vi "Main.vi"() -> ()   [LabVIEW 2013]
uses:
  <vilib>/Utility/miscctls.llb/LVFontTypeDef.ctl
  <vilib>/Utility/error.llb/DialogType.ctl
panel:
  out "Error BuvVIctrl":string[](array[string])
  in  "Num of Buvs":u8
  out "BuvCtrlVI_VIRef":refnum<vi>[](array[refnum])
  out "BuvNameArr":string[](array[string])
  out "Buv IP":string[](array[string])
  out "Buv con ID":refnum<k5>
  out "LoadPhase":bool
  in  "Tab Control":enum32{"ПОСТОЯННОГО ТОКА", "ИМПУЛЬСНЫЕ"}(tab)
  in  "List of channels":i32(listbox)
  in  "ReadFromFile":bool
  in  "WriteToFile":bool
  out "Дата":string
  out "Время":string
  in  "Comm. current inc":dbl=0.5 caption="А" min=0.0 max=72.0 step=0.25
  in  "Common curr. dec":bool
  in  "Common curr. inc":bool
  in  "ConnectAll":bool
  in  "DisconnectAll":bool
  in  "Set Output ON All":bool caption="ВЫХОДЫ ИСТОЧНИКОВ"
  out "текущий ист.":u8
  in  "SetCurrent":dbl min=0.0 max=72.0 step=0.1 format="%#.1g"
  in  "SetVoltage":dbl min=0.0 max=30.0 step=0.1 format="%#.1g"
  in  "SetCurrentB":bool
  in  "SetVoltageB":bool
  in  "SetOutputOffB":bool
  in  "SetOutputOnB":bool
  in  "ConnectChannel":bool
  in  "DisconnectChannel":bool
  in  "WriteToFile Buv":bool
  in  "ReadFromFile Buv":bool
  in  "NewBuvName":string caption="Имя"
  in  "NewBuvIP":string="172.16.21.xx" caption="IP"
  in  "DeleteBuv":bool caption="Удалить БУВ"
  in  "Quit":bool=TRUE
  in  "AddNewBuv":bool caption="Добавить БУВ"
  out "message event":string=" INSTRUCTIONS:\r\rNormal Use:  When using subVIs that incorporate the error in/error out (or error I/O) structure, place this handler where you want to inform the user of an error, typically at the end of the I/O data path, as the last action of the program.  If the error in error? is ERROR, the handler creates a message describing the error and its source.  If the type of dialog = 1 (default), the message is displayed to the user, who can only acknowedge it.  If the type = 2, the user can acknowledge the message or abort execution; aborting a program with active I/O is not recommended.  If the type = 0, no message is displayed; this is used to process the error programmatically, and the error out cluster elements are wired to individual terminals for that reason.  \r\rOther Use:\n\r\nlocal testing.  To test the error code of a subVI or function that does not have the error I/O structure, you can wire its error code and a source string to the local error code and error source inputs.  If error in error? indicates no error and error code is not equal to 0, the local code and source are substituted for the error in values, and error? is set TRUE (ERROR)."
  out "message upd":string=" INSTRUCTIONS:\r\rNormal Use:  When using subVIs that incorporate the error in/error out (or error I/O) structure, place this handler where you want to inform the user of an error, typically at the end of the I/O data path, as the last action of the program.  If the error in error? is ERROR, the handler creates a message describing the error and its source.  If the type of dialog = 1 (default), the message is displayed to the user, who can only acknowedge it.  If the type = 2, the user can acknowledge the message or abort execution; aborting a program with active I/O is not recommended.  If the type = 0, no message is displayed; this is used to process the error programmatically, and the error out cluster elements are wired to individual terminals for that reason.  \r\rOther Use:\n\r\nlocal testing.  To test the error code of a subVI or function that does not have the error I/O structure, you can wire its error code and a source string to the local error code and error source inputs.  If error in error? indicates no error and error code is not equal to 0, the local code and source are substituted for the error in values, and error? is set TRUE (ERROR)."
  in  "List of LU buw":i32(listbox)
  in  "SetCurrentAll":bool
  in  "SetVoltageAll":bool
  in  "Comm. voltage %":dbl caption="%" min=0.0 max=100.0 step=0.5
  in  "Common volt. dec":bool
  in  "Common volt. inc":bool
  in  "DeleteChannel":bool
  in  "AddChannel":bool
  out "CURRENTSET":dbl[](array[numeric])
  out "NAME":string[](array[string])
  out "ADRESS":string[](array[string])
  out "Measure_VI":refnum<vi>[](array[refnum])
  # "ЛИНЗЫ ЖЕСТКОЙ ФОКУСИРОВКИ"
  # "ВСЕ ИСТОЧНИКИ"
  # "ИСТОЧНИК №_"
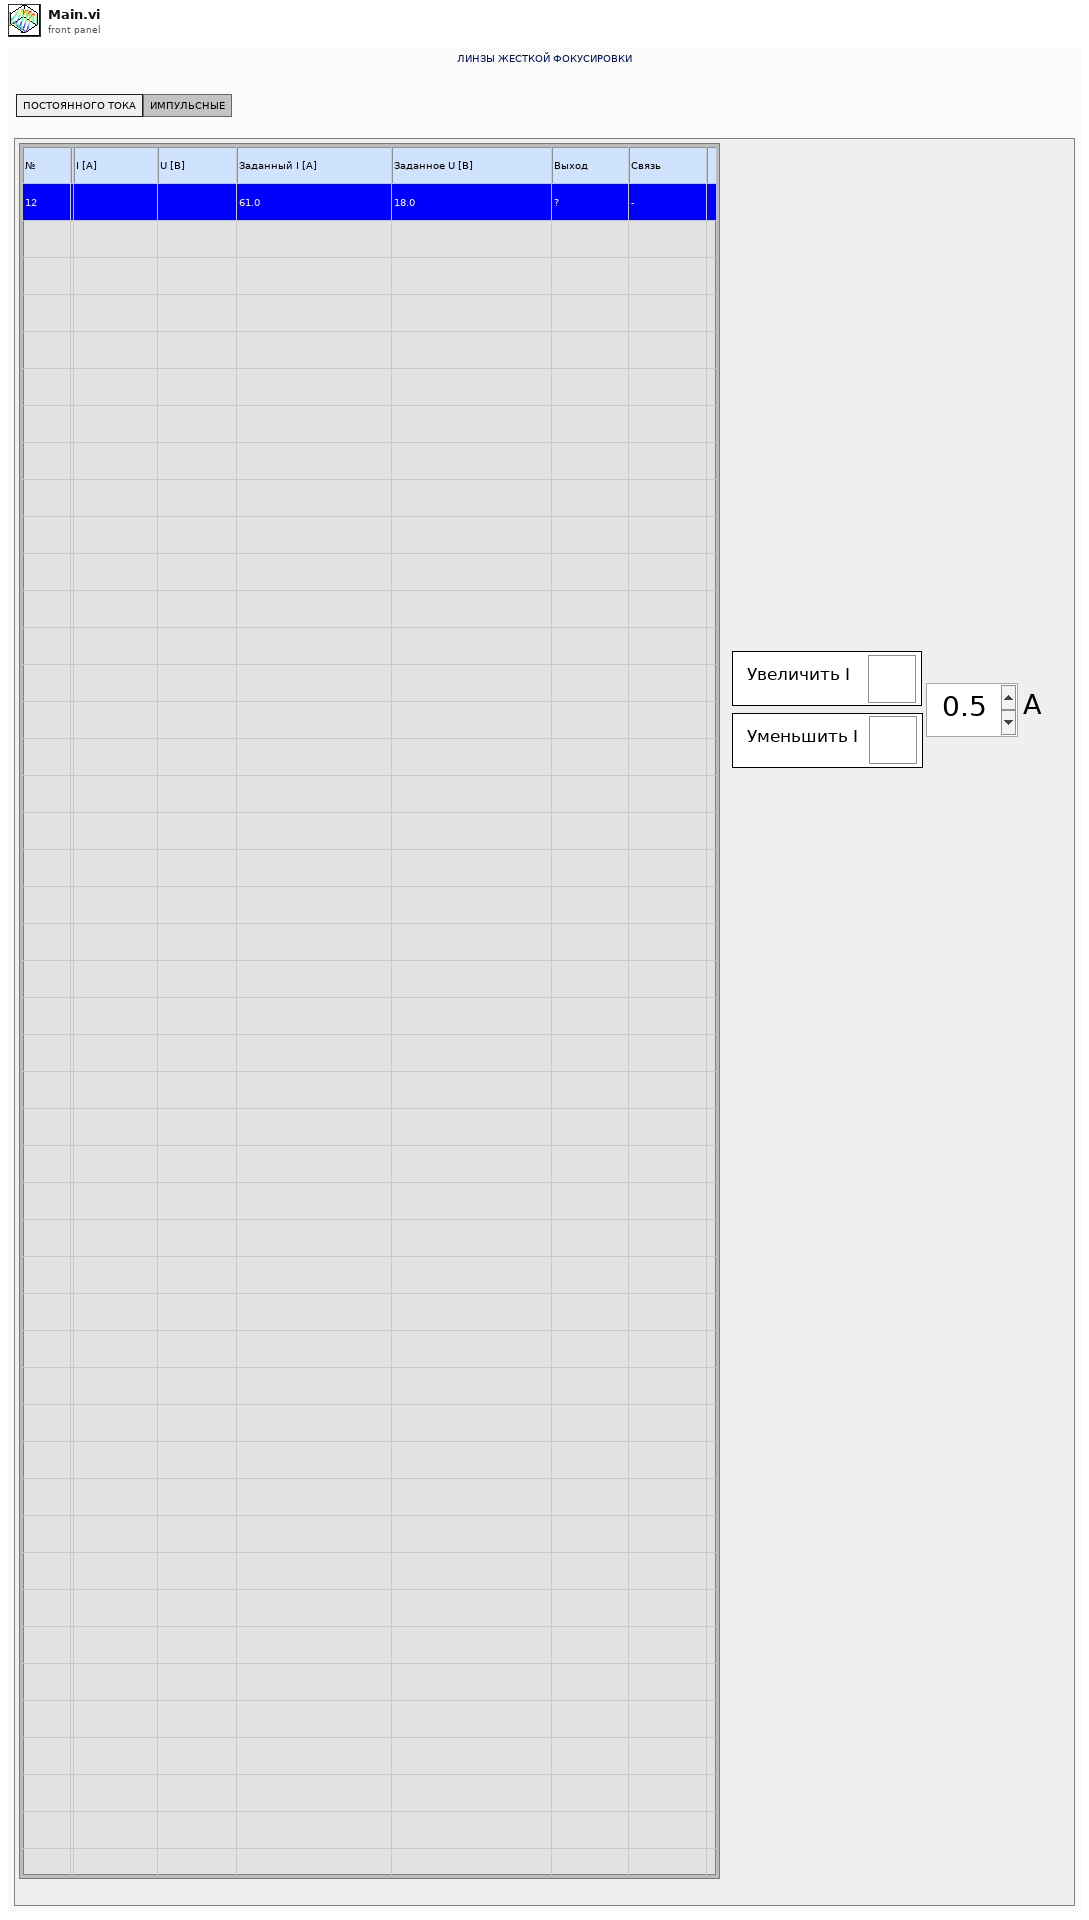
[diagram p1: front panel]
types:
  T1 = enum8{"Enabled", "Disabled", "Disabled and Grayed Out"}
  T2 = enum16{"open", "replace", "create", "open or create", "replace or create", "replace or create with confirmation"}
  T3 = typedef "DialogType.ctl" = u16
  T4 = typedef "LVFontTypeDef.ctl" = cluster{"Font Name":string, "Size":u16, "Bold":bool, "Italic":bool, "Underline":bool, "Strikeout":bool, "Color":u32}
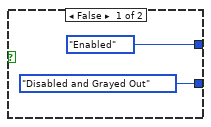
[diagram p3: hidden frame]
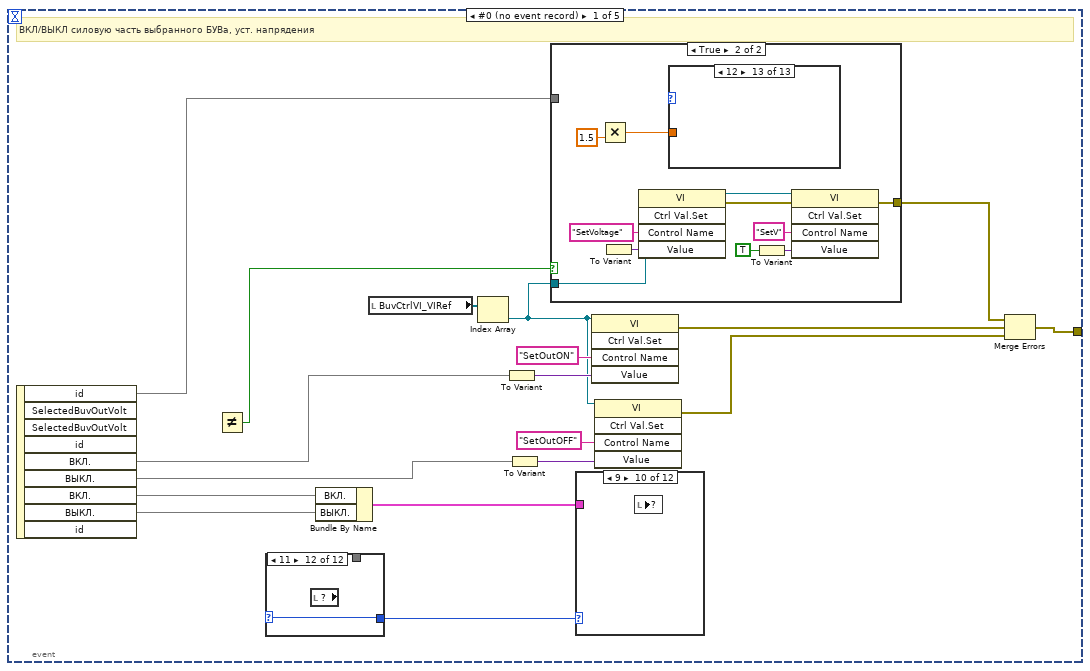
[diagram p4: hidden frame]
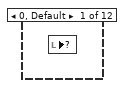
[diagram p5: hidden frame]
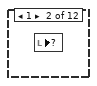
[diagram p6: hidden frame]
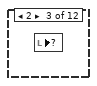
[diagram p7: hidden frame]
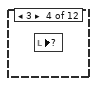
[diagram p8: hidden frame]
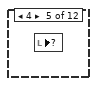
[diagram p9: hidden frame]
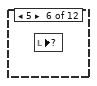
[diagram p10: hidden frame]
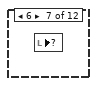
[diagram p11: hidden frame]
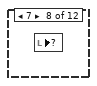
[diagram p12: hidden frame]
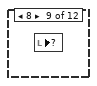
[diagram p13: hidden frame]
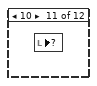
[diagram p14: hidden frame]
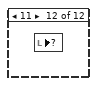
[diagram p15: hidden frame]
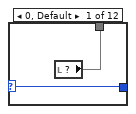
[diagram p16: hidden frame]
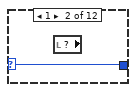
[diagram p17: hidden frame]
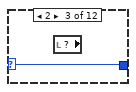
[diagram p18: hidden frame]
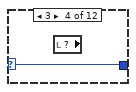
[diagram p19: hidden frame]
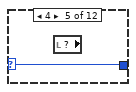
[diagram p20: hidden frame]
diagram:
  w2 = string[] [] ("GlobalInAdress")
  w5 = string[] [] ("GlobalInAdress")
  (unwired) T1."Enabled" ("Disabled")
  w21 = u8 0 ("Disabled")
  w6 = FALSE ("SetOutputOnB")
  w23 = FALSE ("OK Button")
  n1 = while {
    stop <- FALSE stop-if-true
    n2 = property on="List of channels" class="MCListbox (strict)"() -> ("ItemNames"=w34:string[][])  [unwired: 2 in, 2 out]
    n3 = Get Date/Time String(want seconds? (F)=TRUE) -> (date string=→"Дата":string, time string=→"Время":string)  [unwired: 2 in]
    n4 = Wait Until Next ms Multiple(millisecond multiple=u16 1000) -> ()  [unwired: 1 out]
    n5 = Empty Array?(array=w34) -> (empty?=w33:bool)
    n6 = case shown="True" w33 {
      tunnel: [T1."Enabled" ("Disabled") T1."Disabled and Grayed Out" ("Disabled")] -> w28
      frame False {
      }
      frame True {
      }
    }
    n7 = property on="Common curr. inc" class="Bool (strict)"("DisabledEnum"=w28) -> ()  [unwired: 2 in, 2 out]
    n8 = property on="Common curr. dec" class="Bool (strict)"("DisabledEnum"=w28) -> ()  [unwired: 2 in, 2 out]
    n9 = property on="Set Output ON All" class="Bool (strict)"("DisabledEnum"=w28) -> ()  [unwired: 2 in, 2 out]
    n10 = property on="Common volt. inc" class="Bool (strict)"("DisabledEnum"=w28) -> ()  [unwired: 2 in, 2 out]
    n11 = property on="DisconnectAll" class="Bool (strict)"("DisabledEnum"=w28) -> ()  [unwired: 2 in, 2 out]
    n12 = property on="SetVoltageB" class="Bool (strict)"("DisabledEnum"=w28) -> ()  [unwired: 2 in, 2 out]
    n13 = property on="ConnectChannel" class="Bool (strict)"("DisabledEnum"=w28) -> ()  [unwired: 2 in, 2 out]
    n14 = property on="SetOutputOnB" class="Bool (strict)"("DisabledEnum"=w28) -> ()  [unwired: 2 in, 2 out]
    n15 = property on="DisconnectChannel" class="Bool (strict)"("DisabledEnum"=w28) -> ()  [unwired: 2 in, 2 out]
    n16 = property on="SetOutputOffB" class="Bool (strict)"("DisabledEnum"=w28) -> ()  [unwired: 2 in, 2 out]
    n17 = property on="ConnectAll" class="Bool (strict)"("DisabledEnum"=w28) -> ()  [unwired: 2 in, 2 out]
    n18 = property on="SetCurrentB" class="Bool (strict)"("DisabledEnum"=w28) -> ()  [unwired: 2 in, 2 out]
  }
  n19 = while {
    stop <- FALSE stop-if-true
    n20 = property on="AddChannel" class="Bool (strict)"() -> ("Disabled"=w45:u8)  [unwired: 2 in, 2 out]
    n21 = Wait Until Next ms Multiple(millisecond multiple=u32 50) -> ()  [unwired: 1 out]
    n22 = local read "Quit"() -> (w43:bool)
    n23 = Not(x=w43) -> (.not. x?=w42:bool)
    n24 = Equal?(x=w45, y=u8 0) -> (x = y?=w41:bool)
    n25 = And(x=w42, y=w41) -> (x .and. y?=w40:bool)
    n26 = case shown="True" w40 {
      frame False {
      }
      frame True {
        w51 = string[] [] ("GlobalInAdress")
        n27 = local read "Measure_VI"() -> (w58:refnum<vi>[])
        n28 = Array Size(array=w58) -> (size(s)=w50:i32)
        n29 = for {
          N: w50 -> [_]
          tunnel: w58 -> [w121]
          shift-right: [w63] -> w49
          shift-left: w51 -> [w60]
          shift-right: [w62] -> w48
          shift-left: w51 -> [w61]
          shift-right: [w112] -> w46
          shift-left: w51 -> [w113]
          shift-right: [w103] -> w47
          shift-left: w51 -> [w108]
          shift-right: [w106] -> w54
          shift-left: w51 -> [w88]
          shift-right: [w101] -> w53
          shift-left: w51 -> [w102]
          i -> [w84]
          w100 = "" ("Control Name")
          n30 = Index Array(array=w121, index=w84) -> (element=w87:refnum<vi>)
          n31 = invoke on="Invoke Node" class="VI" method="Ctrl Val.Get"(reference=w87, "Control Name"="SetVoltageStr") -> (error out=w95:errorcluster, "Get Control Value Variant"=w111:variant)  [unwired: 2 in, 2 out]
          n32 = invoke class="VI" method="Ctrl Val.Get"(reference=w87, "Control Name"="SetCurrentStr") -> (error out=w94:errorcluster, "Get Control Value Variant"=w110:variant)  [unwired: 2 in, 2 out]
          n33 = invoke class="VI" method="Ctrl Val.Get"(reference=w87, "Control Name"="Error") -> (error out=w83:errorcluster, "Get Control Value Variant"=w89:variant)  [unwired: 2 in, 2 out]
          n34 = invoke class="VI" method="Ctrl Val.Get"(reference=w87, "Control Name"="GetCurrent") -> (error out=w97:errorcluster, "Get Control Value Variant"=w118:variant)  [unwired: 2 in, 2 out]
          n35 = invoke class="VI" method="Ctrl Val.Get"(reference=w87, "Control Name"="GetVoltage") -> (error out=w96:errorcluster, "Get Control Value Variant"=w119:variant)  [unwired: 2 in, 2 out]
          n36 = invoke class="VI" method="Ctrl Val.Get"(reference=w87, "Control Name"="Output") -> (error out=w93:errorcluster, "Get Control Value Variant"=w104:variant)  [unwired: 2 in, 2 out]
          n37 = Variant To Data(type=w100, Variant=w111) -> (data=w65:string)  [unwired: 1 in, 1 out]
          n38 = Variant To Data(type=w100, Variant=w110) -> (data=w70:string)  [unwired: 1 in, 1 out]
          n39 = Merge Errors(w83, w97, w96, w95) -> (w92:errorcluster)
          n40 = Variant To Data(type=w100, Variant=w118) -> (data=w115:string)  [unwired: 1 in, 1 out]
          n41 = Variant To Data(type=w100, Variant=w119) -> (data=w116:string)  [unwired: 1 in, 1 out]
          n42 = Variant To Data "Out"(type=w100, Variant=w104) -> (data=w90:string)  [unwired: 1 in, 1 out]
          n43 = Merge Errors(w94, w93) -> (w91:errorcluster)
          n44 = String Length(string=w65) -> (length=w66:i32)
          n45 = String Length(string=w70) -> (length=w73:i32)
          n46 = Variant To Data(type=FALSE, Variant=w89) -> (data=w59:bool)  [unwired: 1 in, 1 out]
          n47 = case shown="False" w59 {
            tunnel: w87 -> [_ w175]
            tunnel: w84 -> [w162 w168]
            tunnel: [w161 w166] -> w80
            frame False {
              n48 = Bundle(w162, "milliseconds to wait"=8) -> (w163:cluster{i32, "milliseconds to wait":i32})  [unwired: 1 in]
              n49 = property on="error" class="MCListbox (strict)"("ActiveCell"=w163, "CellBG"=u32 16777225) -> (error out=w161:errorcluster)  [unwired: 2 in, 1 out]
            }
            frame True {
              n50 = disable-structure shown="Enabled" {
                disable-tunnel: w175 -> [w191 w197]
                disable-tunnel: [w188 _] -> w171
                disable-tunnel: [w186 w197] -> w170
                disable-tunnel: [w184 _] -> w169
                disable-tunnel: w168 -> [w183 w198]
                disable-tunnel: [w182 w198] -> w167
                frame Disabled {
                  w185 = "Connect" ("Control Name")
                  n51 = invoke class="VI" method="Ctrl Val.Set"(reference=w191, "Control Name"=w185, "Value"=FALSE ("OK Button")) -> (reference out=w187:refnum<vi>, error out=w189:errorcluster)  [unwired: 2 in, 3 out]
                  n52 = flat-sequence {
                    tunnel: w189 -> [w196]
                    tunnel: [w196] -> w188
                    tunnel: w187 -> [w194]
                    tunnel: [w194] -> w186
                    tunnel: w185 -> [w193]
                    tunnel: [w193] -> w184
                    tunnel: w183 -> [w192]
                    tunnel: [w192] -> w182
                    frame #0 {
                      n53 = Wait (ms)(milliseconds to wait=u32 2000) -> ()  [unwired: 1 out]
                    }
                  }
                }
                frame Enabled {
                }
              }
              n54 = disable-structure shown="Enabled" {
                disable-tunnel: w171 -> [w179 w181]
                disable-tunnel: w170 -> [w178 _]
                disable-tunnel: w169 -> [w177 _]
                disable-tunnel: [w176 w181] -> w166
                frame Disabled {
                  n55 = invoke class="VI" method="Ctrl Val.Set"(reference=w178, error in=w179, "Control Name"=w177, "Value"=TRUE ("OK Button")) -> (error out=w176:errorcluster)  [unwired: 1 in, 4 out]
                }
                frame Enabled {
                }
              }
              n56 = Bundle(w167, "milliseconds to wait"=8) -> (w172:cluster{i32, "milliseconds to wait":i32})  [unwired: 1 in]
              n57 = property on="error" class="MCListbox (strict)"("ActiveCell"=w172, "CellBG"=u32 16711680) -> ()  [unwired: 2 in, 2 out]
            }
          }
          n58 = case shown="6, Default" w66 {
            tunnel: [4 ("milliseconds to wait") 5 ("milliseconds to wait")] -> w67
            tunnel: [0 ("milliseconds to wait") 0 ("milliseconds to wait")] -> w68
            frame 6, Default {
            }
            frame 7 {
            }
          }
          n59 = case shown="7" w73 {
            tunnel: [4 ("milliseconds to wait") 5 ("milliseconds to wait")] -> w72
            tunnel: [0 ("milliseconds to wait") 0 ("milliseconds to wait")] -> w71
            frame 6, Default {
            }
            frame 7 {
            }
          }
          n60 = Build Array (concatenate)(w60, w115) -> (w63:string[])
          n61 = Build Array (concatenate)(w61, w116) -> (w62:string[])
          n62 = Merge Errors(w92, w91, w80) -> (w86:errorcluster)
          n63 = call <vilib>:"General Error Handler.vi"("type of dialog (OK msg:1)"=u32 0 ("milliseconds to wait"), "error in (no error)"=w86) -> ()  [unwired: 9 in, 5 out]
          n64 = case shown="\"0\"" w90 {
            tunnel: ["+" ("Control Name") "" ("Control Name") "-" ("Control Name")] -> w82
            tunnel: w84 -> [w130 w135 w140]
            frame "1" {
              n65 = Bundle(w130, "milliseconds to wait"=6) -> (w132:cluster{i32, "milliseconds to wait":i32})  [unwired: 1 in]
              n66 = property on="out" class="MCListbox (strict)"("ActiveCell"=w132, "CellBG"=u32 5895331) -> ()  [unwired: 2 in, 2 out]
            }
            frame Default {
              n67 = Bundle(w135, "milliseconds to wait"=6) -> (w137:cluster{i32, "milliseconds to wait":i32})  [unwired: 1 in]
              n68 = property on="out" class="MCListbox (strict)"("ActiveCell"=w137, "CellBG"=u32 16777225) -> ()  [unwired: 2 in, 2 out]
            }
            frame "0" {
              n69 = Bundle(w140, "milliseconds to wait"=6) -> (w142:cluster{i32, "milliseconds to wait":i32})  [unwired: 1 in]
              n70 = property on="out" class="MCListbox (strict)"("ActiveCell"=w142, "CellBG"=u32 13816530) -> ()  [unwired: 2 in, 2 out]
            }
          }
          n71 = String Subset(string=w65, offset (0)=w68, length (rest)=w67) -> (substring=w64:string)
          n72 = String Subset(string=w70, offset (0)=w71, length (rest)=w72) -> (substring=w69:string)
          n73 = case shown="False" w59 {
            tunnel: ["+" ("Control Name") "-" ("Control Name")] -> w107
            tunnel: w84 -> [w146 w153]
            tunnel: w82 -> [w145 _]
            tunnel: [w145 "?" ("Control Name")] -> w81
            frame False {
              n74 = Bundle(w146, "milliseconds to wait"=7) -> (w148:cluster{i32, "milliseconds to wait":i32})  [unwired: 1 in]
              n75 = property on="active" class="MCListbox (strict)"("ActiveCell"=w148, "CellBG"=u32 5895331) -> ()  [unwired: 2 in, 2 out]
            }
            frame True {
              n76 = Bundle(w153, "milliseconds to wait"=7) -> (w159:cluster{i32, "milliseconds to wait":i32})  [unwired: 1 in]
              n77 = property on="active" class="MCListbox (strict)"("ActiveCell"=w159, "CellBG"=u32 14869218) -> (error out=w154:errorcluster)  [unwired: 2 in, 1 out]
              n78 = Bundle(w153, "milliseconds to wait"=6) -> (w152:cluster{i32, "milliseconds to wait":i32})  [unwired: 1 in]
              n79 = property on="out" class="MCListbox (strict)"(error in=w154, "ActiveCell"=w152, "CellBG"=u32 14869218) -> ()  [unwired: 1 in, 2 out]
            }
          }
          n80 = Search and Replace String(input string=w64, search string=",", replace string="." ("replace string (\"\")")) -> (result string=w77:string)  [unwired: 5 in, 3 out]
          n81 = Search and Replace String(input string=w69, search string=",", replace string="." ("replace string (\"\")")) -> (result string=w75:string)  [unwired: 5 in, 3 out]
          n82 = Build Array (concatenate)(w108, w75) -> (w103:string[])
          n83 = Build Array (concatenate)(w113, w77) -> (w112:string[])
          n84 = Build Array (concatenate)(w102, w81) -> (w101:string[])
          n85 = Build Array (concatenate)(w88, w107) -> (w106:string[])
        }
        n86 = local read "ADRESS"() -> (w56:string[])
        n87 = local read "NAME"() -> (w55:string[])
        n88 = Build Array(w55, w56, w49, w48, w47, w46, w53, w54) -> (w57:string[][])
        n89 = Transpose 2D Array(2D array=w57) -> (transposed array=w52:string[][])
        n90 = property on="List of channels" class="MCListbox (strict)"("ItemNames"=w52) -> ()  [unwired: 2 in, 2 out]
      }
    }
  }
  n91 = while {
    stop <- FALSE stop-if-true
    n92 = event shown="[15] \"ReadFromFile\": Value Change" {
      selector: _ -> [_ _ _ _ _ _ _ _ _ _ _ _ _ _ _ _ _ _]
      dyn-events: _ -> [_ _ _ _ _ _ _ _ _ _ _ _ _ _ _ _ _ _]
      timeout: _ -> [_ _ _ _ _ _ _ _ _ _ _ _ _ _ _ _ _ _]
      tunnel: [_ _ w269 w285 w301 w342 w383 w398 w429 w445 w461 w478 w499 w522 w540 w591 w669 w692] -> w200
      event "List of channels": Mouse Down {
        # "Работа с выбранным источником"
        n93 = event-data() -> ()  [unwired: 2 out]
        n94 = property on="List of channels" class="MCListbox (strict)"() -> ("ItemNames"=w206:string[][])  [unwired: 2 in, 2 out]
        n95 = property on="List of channels" class="MCListbox (strict)"() -> ("Value"=w205:i32)  [unwired: 2 in, 2 out]
        n96 = Index Array(array=w206, index (row)=w205) -> (element=w204:string[])  [unwired: 1 in]
        n97 = Empty Array?(array=w204) -> (empty?=w203:bool)
        n98 = case shown="False" w203 {
          tunnel: w204 -> [w207 _]
          frame False {
            n99 = flat-sequence {
              tunnel: w207 -> [w213]
              tunnel: [w213] -> w208
              tunnel: w208 -> [w226]
              frame #0 {
                n100 = Index Array(array=w213, index=0) -> (element=w216:string)
                n101 = Index Array(array=w213, index=7) -> (element=w214:string)
                n102 = case shown="\"-\", Default" w214 {
                  tunnel: [T1."Enabled" ("Disabled") T1."Disabled and Grayed Out" ("Disabled")] -> w209
                  tunnel: [w220 w222] -> w210
                  tunnel: [w220 w222] -> w212
                  tunnel: [w220 w222] -> w211
                  frame "-", Default {
                    w220 = T1."Disabled and Grayed Out" ("Disabled")
                  }
                  frame "+" {
                    w222 = T1."Enabled" ("Disabled")
                    # "соединение с ист."
                  }
                }
                n103 = Scan From String(format string="%f", input string=w216) -> (output 1=→"текущий ист.":u8)  [unwired: 3 in, 3 out]
                n104 = property on="DisconnectAll" class="Bool (strict)"("DisabledEnum"=w210) -> ()  [unwired: 2 in, 2 out]
                n105 = property on="DisconnectChannel" class="Bool (strict)"("DisabledEnum"=w210) -> ()  [unwired: 2 in, 2 out]
                n106 = property on="SetOutputOffB" class="Bool (strict)"("DisabledEnum"=w212) -> ()  [unwired: 2 in, 2 out]
                n107 = property on="SetOutputOnB" class="Bool (strict)"("DisabledEnum"=w211) -> ()  [unwired: 2 in, 2 out]
                n108 = property on="ConnectChannel" class="Bool (strict)"("DisabledEnum"=w209) -> ()  [unwired: 2 in, 2 out]
                n109 = property on="ConnectAll" class="Bool (strict)"("DisabledEnum"=w209) -> ()  [unwired: 2 in, 2 out]
              }
              frame #1 {
                n110 = Index Array(array=w226, index=5) -> (element=w231:string)
                n111 = Index Array(array=w226, index=6) -> (element=w234:string)
                n112 = Index Array(array=w226, index=4) -> (element=w228:string)
                n113 = case shown="\"-\", Default" w234 {
                  tunnel: [T1."Enabled" ("Disabled") T1."Disabled and Grayed Out" ("Disabled") w241] -> w235
                  tunnel: [T1."Disabled and Grayed Out" ("Disabled") T1."Enabled" ("Disabled") w241] -> w236
                  frame "-", Default {
                  }
                  frame "+" {
                  }
                  frame "?" {
                    w241 = T1."Disabled and Grayed Out" ("Disabled")
                  }
                }
                n114 = Scan From String(format string="%f", input string=w231) -> (output 1=w224:dbl)  [unwired: 3 in, 3 out]
                n115 = Scan From String(format string="%f", input string=w228) -> (output 1=w225:dbl)  [unwired: 3 in, 3 out]
                n116 = local write "SetVoltage"(w224) -> ()
                n117 = local write "SetCurrent"(w225) -> ()
                n118 = property on="SetOutputOffB" class="Bool (strict)"("DisabledEnum"=w236) -> ()  [unwired: 2 in, 2 out]
                n119 = property on="SetOutputOnB" class="Bool (strict)"("DisabledEnum"=w235) -> ()  [unwired: 2 in, 2 out]
              }
            }
          }
          frame True {
          }
        }
      }
      event Panel Close? {
        n120 = event-data() -> ()  [unwired: 5 out]
        n121 = Two Button Dialog(message="Вы уверены, что хотите закрыть программу?", 1:"Нет" ("F button name (\"Cancel\")"), 2:"Да" ("T button name (\"OK\")")) -> (T button?=w245:bool)
        n122 = case shown="True" w245 {
          frame False {
          }
          frame True {
            n123 = disable-structure shown="Disabled" {
              frame Disabled {
                n124 = local read item#-1() -> (w255)
                n125 = TCP Close Connection(connection ID=w255) -> ()  [unwired: 2 in, 2 out]
              }
              frame Enabled {
              }
            }
            n126 = local read "Measure_VI"() -> (w247:refnum<vi>[])
            n127 = Array Size(array=w247) -> (size(s)=w246:i32)
            n128 = for {
              N: w246 -> [_]
              tunnel: w247 -> [w265]
              tunnel: [w263] -> w254 mode=indexing
              i -> [w266]
              n129 = Index Array(array=w265, index=w266) -> (element=w264:refnum<vi>)
              n130 = invoke class="VI" method="Ctrl Val.Set"(reference=w264, "Control Name"="Connect", "Value"=FALSE) -> (error out=w263:errorcluster)  [unwired: 2 in, 4 out]
            }
            n131 = flat-sequence {
              tunnel: [w257] -> w253
              tunnel: w254 -> [w257]
              frame #0 {
                n132 = Wait (ms)(milliseconds to wait=u32 1000) -> ()  [unwired: 1 out]
              }
            }
            n133 = local read "Measure_VI"() -> (w248:refnum<vi>[])
            n134 = Array Size(array=w248) -> (size(s)=w249:i32)
            n135 = for {
              N: w249 -> [_]
              tunnel: w248 -> [w261]
              tunnel: [w259] -> w250 mode=indexing
              tunnel: w253 -> [w258] mode=indexing
              i -> [w262]
              n136 = Index Array(array=w261, index=w262) -> (element=w260:refnum<vi>)
              n137 = invoke class="VI" method="Abort VI"(reference=w260, error in=w258) -> (error out=w259:errorcluster)  [unwired: 1 in, 2 out]
            }
            n138 = Merge Errors(w250) -> (w251:errorcluster)
            n139 = call <vilib>:"General Error Handler.vi"("type of dialog (OK msg:1)"=u32 0 ("milliseconds to wait"), "error in (no error)"=w251) -> ()  [unwired: 9 in, 5 out]
          }
        }
        n140 = event-data() -> ()  [unwired: 2 in, 1 out]
      }
      event "SetVoltageAll": Value Change {
        n141 = event-data() -> ()  [unwired: 7 out]
        n142 = flat-sequence {
          tunnel: [w273] -> w271
          tunnel: [w282] -> w270
          tunnel: w271 -> [w282]
          frame #0 {
            w272 = u8 2 ("Disabled")
            n143 = property on="Quit" class="Bool (strict)"("Disabled"=w272) -> ()  [unwired: 2 in, 2 out]
            n144 = property on="AddChannel" class="Bool (strict)"("Disabled"=w272) -> ()  [unwired: 2 in, 2 out]
            n145 = property on="DisconnectChannel" class="Bool (strict)"("Disabled"=w272) -> ()  [unwired: 2 in, 2 out]
            n146 = property on="ConnectAll" class="Bool (strict)"("Disabled"=w272) -> ()  [unwired: 2 in, 2 out]
            n147 = property on="ReadFromFile" class="Bool (strict)"("Disabled"=w272) -> ()  [unwired: 2 in, 2 out]
            n148 = property on="ConnectChannel" class="Bool (strict)"("Disabled"=w272) -> ()  [unwired: 2 in, 2 out]
            n149 = property on="DeleteChannel" class="Bool (strict)"("Disabled"=w272) -> ()  [unwired: 2 in, 2 out]
            n150 = property on="SetVoltageB" class="Bool (strict)"("Disabled"=w272) -> ()  [unwired: 2 in, 2 out]
            n151 = property on="Set Output ON All" class="Bool (strict)"("Disabled"=w272) -> ()  [unwired: 2 in, 2 out]
            n152 = property on="SetOutputOffB" class="Bool (strict)"("Disabled"=w272) -> ()  [unwired: 2 in, 2 out]
            n153 = property on="SetVoltageAll" class="Bool (strict)"("Disabled"=w272) -> ()  [unwired: 2 in, 2 out]
            n154 = property on="SetCurrentAll" class="Bool (strict)"("Disabled"=w272) -> ()  [unwired: 2 in, 2 out]
            n155 = property on="DisconnectAll" class="Bool (strict)"("Disabled"=w272) -> ()  [unwired: 2 in, 2 out]
            n156 = property on="WriteToFile" class="Bool (strict)"("Disabled"=w272) -> ()  [unwired: 2 in, 2 out]
            n157 = property on="SetCurrentB" class="Bool (strict)"("Disabled"=w272) -> ()  [unwired: 2 in, 2 out]
            n158 = property on="SetOutputOnB" class="Bool (strict)"("Disabled"=w272) -> ()  [unwired: 2 in, 2 out]
          }
          frame #1 {
            n159 = local read "Measure_VI"() -> (w275:refnum<vi>[])
            n160 = Array Size(array=w275) -> (size(s)=w274:i32)
            n161 = for {
              N: w274 -> [_]
              tunnel: [w276] -> w273 mode=indexing
              i -> [w278]
              n162 = local read "Measure_VI"() -> (w281:refnum<vi>[])
              n163 = Index Array(array=w281, index=w278) -> (element=w277:refnum<vi>)
              n164 = invoke class="VI" method="Ctrl Val.Set"(reference=w277, "Control Name"="NeedToSetVoltage", "Value"=TRUE ("ConnectChannel")) -> (error out=w276:errorcluster)  [unwired: 2 in, 4 out]
            }
          }
          frame #2 {
            w283 = u8 0 ("Disabled")
            n165 = local write "SetVoltageAll"(FALSE ("SetVoltageAll")) -> ()
            n166 = property on="Quit" class="Bool (strict)"("Disabled"=w283) -> ()  [unwired: 2 in, 2 out]
            n167 = property on="AddChannel" class="Bool (strict)"("Disabled"=w283) -> ()  [unwired: 2 in, 2 out]
            n168 = property on="DisconnectChannel" class="Bool (strict)"("Disabled"=w283) -> ()  [unwired: 2 in, 2 out]
            n169 = property on="ReadFromFile" class="Bool (strict)"("Disabled"=w283) -> ()  [unwired: 2 in, 2 out]
            n170 = property on="ConnectChannel" class="Bool (strict)"("Disabled"=w283) -> ()  [unwired: 2 in, 2 out]
            n171 = property on="DeleteChannel" class="Bool (strict)"("Disabled"=w283) -> ()  [unwired: 2 in, 2 out]
            n172 = property on="WriteToFile" class="Bool (strict)"("Disabled"=w283) -> ()  [unwired: 2 in, 2 out]
            n173 = property on="Set Output ON All" class="Bool (strict)"("Disabled"=w283) -> ()  [unwired: 2 in, 2 out]
            n174 = property on="SetCurrentB" class="Bool (strict)"("Disabled"=w283) -> ()  [unwired: 2 in, 2 out]
            n175 = property on="ConnectAll" class="Bool (strict)"("Disabled"=w283) -> ()  [unwired: 2 in, 2 out]
            n176 = property on="SetOutputOnB" class="Bool (strict)"("Disabled"=w283) -> ()  [unwired: 2 in, 2 out]
            n177 = property on="SetVoltageB" class="Bool (strict)"("Disabled"=w283) -> ()  [unwired: 2 in, 2 out]
            n178 = property on="SetOutputOffB" class="Bool (strict)"("Disabled"=w283) -> ()  [unwired: 2 in, 2 out]
            n179 = property on="SetVoltageAll" class="Bool (strict)"("Disabled"=w283) -> ()  [unwired: 2 in, 2 out]
            n180 = property on="SetCurrentAll" class="Bool (strict)"("Disabled"=w283) -> ()  [unwired: 2 in, 2 out]
            n181 = property on="DisconnectAll" class="Bool (strict)"("Disabled"=w283) -> ()  [unwired: 2 in, 2 out]
          }
        }
        n182 = Merge Errors(w270) -> (w269:errorcluster)
      }
      event "SetCurrentAll": Value Change {
        n183 = event-data() -> ()  [unwired: 7 out]
        n184 = flat-sequence {
          tunnel: [w289] -> w287
          tunnel: [w298] -> w286
          tunnel: w287 -> [w298]
          frame #0 {
            w288 = u8 2 ("Disabled")
            n185 = property on="Quit" class="Bool (strict)"("Disabled"=w288) -> ()  [unwired: 2 in, 2 out]
            n186 = property on="AddChannel" class="Bool (strict)"("Disabled"=w288) -> ()  [unwired: 2 in, 2 out]
            n187 = property on="DisconnectChannel" class="Bool (strict)"("Disabled"=w288) -> ()  [unwired: 2 in, 2 out]
            n188 = property on="ConnectAll" class="Bool (strict)"("Disabled"=w288) -> ()  [unwired: 2 in, 2 out]
            n189 = property on="ReadFromFile" class="Bool (strict)"("Disabled"=w288) -> ()  [unwired: 2 in, 2 out]
            n190 = property on="ConnectChannel" class="Bool (strict)"("Disabled"=w288) -> ()  [unwired: 2 in, 2 out]
            n191 = property on="DeleteChannel" class="Bool (strict)"("Disabled"=w288) -> ()  [unwired: 2 in, 2 out]
            n192 = property on="SetOutputOffB" class="Bool (strict)"("Disabled"=w288) -> ()  [unwired: 2 in, 2 out]
            n193 = property on="Set Output ON All" class="Bool (strict)"("Disabled"=w288) -> ()  [unwired: 2 in, 2 out]
            n194 = property on="SetVoltageAll" class="Bool (strict)"("Disabled"=w288) -> ()  [unwired: 2 in, 2 out]
            n195 = property on="SetCurrentAll" class="Bool (strict)"("Disabled"=w288) -> ()  [unwired: 2 in, 2 out]
            n196 = property on="DisconnectAll" class="Bool (strict)"("Disabled"=w288) -> ()  [unwired: 2 in, 2 out]
            n197 = property on="WriteToFile" class="Bool (strict)"("Disabled"=w288) -> ()  [unwired: 2 in, 2 out]
            n198 = property on="SetCurrentB" class="Bool (strict)"("Disabled"=w288) -> ()  [unwired: 2 in, 2 out]
            n199 = property on="SetOutputOnB" class="Bool (strict)"("Disabled"=w288) -> ()  [unwired: 2 in, 2 out]
            n200 = property on="SetVoltageB" class="Bool (strict)"("Disabled"=w288) -> ()  [unwired: 2 in, 2 out]
          }
          frame #1 {
            n201 = local read "Measure_VI"() -> (w291:refnum<vi>[])
            n202 = Array Size(array=w291) -> (size(s)=w290:i32)
            n203 = for {
              N: w290 -> [_]
              tunnel: [w292] -> w289 mode=indexing
              i -> [w294]
              n204 = local read "Measure_VI"() -> (w297:refnum<vi>[])
              n205 = Index Array(array=w297, index=w294) -> (element=w293:refnum<vi>)
              n206 = invoke class="VI" method="Ctrl Val.Set"(reference=w293, "Control Name"="NeedToSetCurrent", "Value"=TRUE ("ConnectChannel")) -> (error out=w292:errorcluster)  [unwired: 2 in, 4 out]
            }
          }
          frame #2 {
            w299 = u8 0 ("Disabled")
            n207 = local write "SetCurrentAll"(FALSE ("SetVoltageAll")) -> ()
            n208 = property on="Quit" class="Bool (strict)"("Disabled"=w299) -> ()  [unwired: 2 in, 2 out]
            n209 = property on="AddChannel" class="Bool (strict)"("Disabled"=w299) -> ()  [unwired: 2 in, 2 out]
            n210 = property on="DisconnectChannel" class="Bool (strict)"("Disabled"=w299) -> ()  [unwired: 2 in, 2 out]
            n211 = property on="ReadFromFile" class="Bool (strict)"("Disabled"=w299) -> ()  [unwired: 2 in, 2 out]
            n212 = property on="ConnectChannel" class="Bool (strict)"("Disabled"=w299) -> ()  [unwired: 2 in, 2 out]
            n213 = property on="DeleteChannel" class="Bool (strict)"("Disabled"=w299) -> ()  [unwired: 2 in, 2 out]
            n214 = property on="WriteToFile" class="Bool (strict)"("Disabled"=w299) -> ()  [unwired: 2 in, 2 out]
            n215 = property on="Set Output ON All" class="Bool (strict)"("Disabled"=w299) -> ()  [unwired: 2 in, 2 out]
            n216 = property on="SetCurrentB" class="Bool (strict)"("Disabled"=w299) -> ()  [unwired: 2 in, 2 out]
            n217 = property on="ConnectAll" class="Bool (strict)"("Disabled"=w299) -> ()  [unwired: 2 in, 2 out]
            n218 = property on="SetOutputOnB" class="Bool (strict)"("Disabled"=w299) -> ()  [unwired: 2 in, 2 out]
            n219 = property on="SetVoltageB" class="Bool (strict)"("Disabled"=w299) -> ()  [unwired: 2 in, 2 out]
            n220 = property on="SetOutputOffB" class="Bool (strict)"("Disabled"=w299) -> ()  [unwired: 2 in, 2 out]
            n221 = property on="SetVoltageAll" class="Bool (strict)"("Disabled"=w299) -> ()  [unwired: 2 in, 2 out]
            n222 = property on="SetCurrentAll" class="Bool (strict)"("Disabled"=w299) -> ()  [unwired: 2 in, 2 out]
            n223 = property on="DisconnectAll" class="Bool (strict)"("Disabled"=w299) -> ()  [unwired: 2 in, 2 out]
          }
        }
        n224 = Merge Errors(w286) -> (w285:errorcluster)
      }
      event "Common curr. inc", "Common curr. dec": Value Change {
        # "Увелич/уменьшение тока на всех ист"
        n225 = event-data() -> ()  [unwired: 2 out]
        n226 = local read "ADRESS"() -> (w304:string[])
        n227 = Array Size(array=w304) -> (size(s)=w305:i32)
        n228 = for {
          N: w305 -> [_]
          tunnel: [w315] -> w303 mode=indexing
          i -> [w329]
          n229 = local read "Measure_VI"() -> (w332:refnum<vi>[])
          n230 = Index Array(array=w332, index=w329) -> (element=w323:refnum<vi>)
          n231 = invoke class="VI" method="Ctrl Val.Get"(reference=w323, "Control Name"="SetCurrentStr") -> (reference out=w317:refnum<vi>, error out=w327:errorcluster, "Get Control Value Variant"=w331:variant)  [unwired: 2 in, 1 out]
          n232 = Variant To Data(error in=w327, type="" ("Control Name"), Variant=w331) -> (data=w326:string, error out=w325:errorcluster)
          n233 = Scan From String(format string="%f", input string=w326, error in=w325) -> (error out=w316:errorcluster, output 1=w314:dbl)  [unwired: 2 in, 2 out]
          n234 = local read "Common curr. inc"() -> (w313:bool)
          n235 = local read "Common curr. dec"() -> (w311:bool)
          n236 = case shown="True" w313 {
            tunnel: "Comm. current inc" -> [w337 w341]
            tunnel: w314 -> [w338 w340]
            tunnel: [w338 w339] -> w312
            tunnel: [w337 _] -> w310
            frame False {
            }
            frame True {
              n237 = Add(x=w340, y=w341) -> (x+y=w339:dbl)
            }
          }
          n238 = case shown="True" w311 {
            tunnel: w312 -> [w333 w336]
            tunnel: [w333 w335] -> w309
            tunnel: w310 -> [_ w334]
            frame False {
            }
            frame True {
              n239 = Subtract(x=w336, y=w334) -> (x-y=w335:dbl)
            }
          }
          n240 = invoke class="VI" method="Ctrl Val.Set"(reference=w317, error in=w316, "Control Name"="SetCurrent", "Value"=w309) -> (reference out=w319:refnum<vi>, error out=w318:errorcluster)  [unwired: 1 in, 3 out]
          n241 = invoke class="VI" method="Ctrl Val.Set"(reference=w319, error in=w318, "Control Name"="NeedToSetCurrent", "Value"=TRUE ("ConnectChannel")) -> (error out=w315:errorcluster)  [unwired: 1 in, 4 out]
        }
        n242 = Merge Errors(w303) -> (w302:errorcluster)
        n243 = flat-sequence {
          tunnel: w302 -> [w307]
          tunnel: [w307] -> w301
          frame #0 {
            w306 = FALSE ("ConnectChannel")
            n244 = local write "Common curr. inc"(w306) -> ()
            n245 = local write "Common curr. dec"(w306) -> ()
          }
        }
      }
      event "Common volt. inc", "Common volt. dec": Value Change {
        # "Увелич/уменьшение тока на всех ист"
        n246 = event-data() -> ()  [unwired: 2 out]
        n247 = local read "ADRESS"() -> (w345:string[])
        n248 = Array Size(array=w345) -> (size(s)=w346:i32)
        n249 = for {
          N: w346 -> [_]
          tunnel: [w356] -> w344 mode=indexing
          i -> [w370]
          n250 = local read "Measure_VI"() -> (w373:refnum<vi>[])
          n251 = Index Array(array=w373, index=w370) -> (element=w364:refnum<vi>)
          n252 = invoke class="VI" method="Ctrl Val.Get"(reference=w364, "Control Name"="SetVoltageStr") -> (reference out=w358:refnum<vi>, error out=w368:errorcluster, "Get Control Value Variant"=w372:variant)  [unwired: 2 in, 1 out]
          n253 = Variant To Data(error in=w368, type="" ("Control Name"), Variant=w372) -> (data=w367:string, error out=w366:errorcluster)
          n254 = Scan From String(format string="%f", input string=w367, error in=w366) -> (error out=w357:errorcluster, output 1=w355:dbl)  [unwired: 2 in, 2 out]
          n255 = local read "Common volt. inc"() -> (w354:bool)
          n256 = local read "Common volt. dec"() -> (w352:bool)
          n257 = case shown="True" w354 {
            tunnel: "Comm. voltage %" -> [w378 w382]
            tunnel: w355 -> [w379 w381]
            tunnel: [w379 w380] -> w353
            tunnel: [w378 _] -> w351
            frame False {
            }
            frame True {
              n258 = Add(x=w381, y=w382) -> (x+y=w380:dbl)
            }
          }
          n259 = case shown="False" w352 {
            tunnel: w353 -> [w374 w377]
            tunnel: [w374 w376] -> w350
            tunnel: w351 -> [_ w375]
            frame False {
            }
            frame True {
              n260 = Subtract(x=w377, y=w375) -> (x-y=w376:dbl)
            }
          }
          n261 = invoke class="VI" method="Ctrl Val.Set"(reference=w358, error in=w357, "Control Name"="SetVoltage", "Value"=w350) -> (reference out=w360:refnum<vi>, error out=w359:errorcluster)  [unwired: 1 in, 3 out]
          n262 = invoke class="VI" method="Ctrl Val.Set"(reference=w360, error in=w359, "Control Name"="NeedToSetVoltage", "Value"=TRUE ("ConnectChannel")) -> (error out=w356:errorcluster)  [unwired: 1 in, 4 out]
        }
        n263 = Merge Errors(w344) -> (w343:errorcluster)
        n264 = flat-sequence {
          tunnel: w343 -> [w348]
          tunnel: [w348] -> w342
          frame #0 {
            w347 = FALSE ("ConnectChannel")
            n265 = local write "Common volt. inc"(w347) -> ()
            n266 = local write "Common volt. dec"(w347) -> ()
          }
        }
      }
      event "DisconnectChannel": Value Change {
        n267 = event-data() -> ()  [unwired: 7 out]
        n268 = property on="List of channels" class="MCListbox (strict)"() -> ("Value"=w387:i32)  [unwired: 2 in, 2 out]
        n269 = flat-sequence {
          tunnel: w387 -> [w389]
          tunnel: [w389] -> w386
          tunnel: w386 -> [w391]
          tunnel: [w390] -> w384
          tunnel: [w396] -> w385
          tunnel: w384 -> [w396]
          frame #0 {
            w388 = u8 2 ("Disabled")
            n270 = property on="AddChannel" class="Bool (strict)"("Disabled"=w388) -> ()  [unwired: 2 in, 2 out]
            n271 = property on="Set Output ON All" class="Bool (strict)"("Disabled"=w388) -> ()  [unwired: 2 in, 2 out]
            n272 = property on="ConnectAll" class="Bool (strict)"("Disabled"=w388) -> ()  [unwired: 2 in, 2 out]
            n273 = property on="DisconnectChannel" class="Bool (strict)"("Disabled"=w388) -> ()  [unwired: 2 in, 2 out]
            n274 = property on="ReadFromFile" class="Bool (strict)"("Disabled"=w388) -> ()  [unwired: 2 in, 2 out]
            n275 = property on="Quit" class="Bool (strict)"("Disabled"=w388) -> ()  [unwired: 2 in, 2 out]
            n276 = property on="ConnectChannel" class="Bool (strict)"("Disabled"=w388) -> ()  [unwired: 2 in, 2 out]
            n277 = property on="DeleteChannel" class="Bool (strict)"("Disabled"=w388) -> ()  [unwired: 2 in, 2 out]
            n278 = property on="WriteToFile" class="Bool (strict)"("Disabled"=w388) -> ()  [unwired: 2 in, 2 out]
            n279 = property on="SetCurrentB" class="Bool (strict)"("Disabled"=w388) -> ()  [unwired: 2 in, 2 out]
            n280 = property on="SetOutputOnB" class="Bool (strict)"("Disabled"=w388) -> ()  [unwired: 2 in, 2 out]
            n281 = property on="SetVoltageB" class="Bool (strict)"("Disabled"=w388) -> ()  [unwired: 2 in, 2 out]
            n282 = property on="SetOutputOffB" class="Bool (strict)"("Disabled"=w388) -> ()  [unwired: 2 in, 2 out]
            n283 = property on="SetVoltageAll" class="Bool (strict)"("Disabled"=w388) -> ()  [unwired: 2 in, 2 out]
            n284 = property on="SetCurrentAll" class="Bool (strict)"("Disabled"=w388) -> ()  [unwired: 2 in, 2 out]
            n285 = property on="DisconnectAll" class="Bool (strict)"("Disabled"=w388) -> ()  [unwired: 2 in, 2 out]
          }
          frame #1 {
            w392 = FALSE ("OK Button")
            n286 = local write "DisconnectChannel"(w392) -> ()
            n287 = local read "Measure_VI"() -> (w394:refnum<vi>[])
            n288 = Index Array(array=w394, index=w391) -> (element=w393:refnum<vi>)
            n289 = invoke class="VI" method="Ctrl Val.Set"(reference=w393, "Control Name"="Connect", "Value"=w392) -> (error out=w390:errorcluster)  [unwired: 2 in, 4 out]
          }
          frame #2 {
            w397 = u8 0 ("Disabled")
            n290 = property on="AddChannel" class="Bool (strict)"("Disabled"=w397) -> ()  [unwired: 2 in, 2 out]
            n291 = property on="DisconnectChannel" class="Bool (strict)"("Disabled"=w397) -> ()  [unwired: 2 in, 2 out]
            n292 = property on="ConnectAll" class="Bool (strict)"("Disabled"=w397) -> ()  [unwired: 2 in, 2 out]
            n293 = property on="ReadFromFile" class="Bool (strict)"("Disabled"=w397) -> ()  [unwired: 2 in, 2 out]
            n294 = property on="ConnectChannel" class="Bool (strict)"("Disabled"=w397) -> ()  [unwired: 2 in, 2 out]
            n295 = property on="Quit" class="Bool (strict)"("Disabled"=w397) -> ()  [unwired: 2 in, 2 out]
            n296 = property on="DeleteChannel" class="Bool (strict)"("Disabled"=w397) -> ()  [unwired: 2 in, 2 out]
            n297 = property on="SetOutputOffB" class="Bool (strict)"("Disabled"=w397) -> ()  [unwired: 2 in, 2 out]
            n298 = property on="Set Output ON All" class="Bool (strict)"("Disabled"=w397) -> ()  [unwired: 2 in, 2 out]
            n299 = property on="SetVoltageAll" class="Bool (strict)"("Disabled"=w397) -> ()  [unwired: 2 in, 2 out]
            n300 = property on="SetCurrentAll" class="Bool (strict)"("Disabled"=w397) -> ()  [unwired: 2 in, 2 out]
            n301 = property on="DisconnectAll" class="Bool (strict)"("Disabled"=w397) -> ()  [unwired: 2 in, 2 out]
            n302 = property on="WriteToFile" class="Bool (strict)"("Disabled"=w397) -> ()  [unwired: 2 in, 2 out]
            n303 = property on="SetCurrentB" class="Bool (strict)"("Disabled"=w397) -> ()  [unwired: 2 in, 2 out]
            n304 = property on="SetOutputOnB" class="Bool (strict)"("Disabled"=w397) -> ()  [unwired: 2 in, 2 out]
            n305 = property on="SetVoltageB" class="Bool (strict)"("Disabled"=w397) -> ()  [unwired: 2 in, 2 out]
          }
        }
        n306 = Merge Errors(w385) -> (w383:errorcluster)
      }
      event "ConnectChannel": Value Change {
        n307 = event-data() -> ()  [unwired: 7 out]
        n308 = property on="List of channels" class="MCListbox (strict)"() -> ("Value"=w402:i32)  [unwired: 2 in, 2 out]
        n309 = flat-sequence {
          tunnel: w402 -> [w404]
          tunnel: [w404] -> w401
          tunnel: w401 -> [w411]
          tunnel: [w410] -> w399
          tunnel: [w426] -> w400
          tunnel: w399 -> [w426]
          frame #0 {
            w403 = u8 2 ("Disabled")
            n310 = property on="AddChannel" class="Bool (strict)"("Disabled"=w403) -> ()  [unwired: 2 in, 2 out]
            n311 = property on="Set Output ON All" class="Bool (strict)"("Disabled"=w403) -> ()  [unwired: 2 in, 2 out]
            n312 = property on="ConnectAll" class="Bool (strict)"("Disabled"=w403) -> ()  [unwired: 2 in, 2 out]
            n313 = property on="DisconnectChannel" class="Bool (strict)"("Disabled"=w403) -> ()  [unwired: 2 in, 2 out]
            n314 = property on="ReadFromFile" class="Bool (strict)"("Disabled"=w403) -> ()  [unwired: 2 in, 2 out]
            n315 = property on="Quit" class="Bool (strict)"("Disabled"=w403) -> ()  [unwired: 2 in, 2 out]
            n316 = property on="ConnectChannel" class="Bool (strict)"("Disabled"=w403) -> ()  [unwired: 2 in, 2 out]
            n317 = property on="DeleteChannel" class="Bool (strict)"("Disabled"=w403) -> ()  [unwired: 2 in, 2 out]
            n318 = property on="WriteToFile" class="Bool (strict)"("Disabled"=w403) -> ()  [unwired: 2 in, 2 out]
            n319 = property on="SetCurrentB" class="Bool (strict)"("Disabled"=w403) -> ()  [unwired: 2 in, 2 out]
            n320 = property on="SetOutputOnB" class="Bool (strict)"("Disabled"=w403) -> ()  [unwired: 2 in, 2 out]
            n321 = property on="SetVoltageB" class="Bool (strict)"("Disabled"=w403) -> ()  [unwired: 2 in, 2 out]
            n322 = property on="SetOutputOffB" class="Bool (strict)"("Disabled"=w403) -> ()  [unwired: 2 in, 2 out]
            n323 = property on="SetVoltageAll" class="Bool (strict)"("Disabled"=w403) -> ()  [unwired: 2 in, 2 out]
            n324 = property on="SetCurrentAll" class="Bool (strict)"("Disabled"=w403) -> ()  [unwired: 2 in, 2 out]
            n325 = property on="DisconnectAll" class="Bool (strict)"("Disabled"=w403) -> ()  [unwired: 2 in, 2 out]
          }
          frame #1 {
            n326 = local read "Measure_VI"() -> (w412:refnum<vi>[])
            n327 = Index Array(array=w412, index=w411) -> (element=w409:refnum<vi>)
            n328 = flat-sequence {
              tunnel: w409 -> [w415]
              tunnel: [w414] -> w407
              tunnel: [w413] -> w405
              tunnel: [w419] -> w408
              tunnel: w407 -> [w419]
              tunnel: [w418] -> w406
              tunnel: w405 -> [w418]
              tunnel: [w422] -> w410
              tunnel: w408 -> [w423]
              tunnel: w406 -> [w421]
              frame #0 {
                n329 = invoke class="VI" method="Ctrl Val.Set"(reference=w415, "Control Name"="Connect", "Value"=FALSE ("OK Button")) -> (reference out=w414:refnum<vi>, error out=w413:errorcluster)  [unwired: 2 in, 3 out]
              }
              frame #1 {
                n330 = Wait (ms)(milliseconds to wait=u32 1000) -> ()  [unwired: 1 out]
              }
              frame #2 {
                n331 = invoke class="VI" method="Ctrl Val.Set"(reference=w423, error in=w421, "Control Name"="Connect", "Value"=TRUE ("OK Button")) -> (error out=w422:errorcluster)  [unwired: 1 in, 4 out]
              }
            }
          }
          frame #2 {
            w427 = u8 0 ("Disabled")
            n332 = local write "ConnectChannel"(FALSE ("ConnectChannel")) -> ()
            n333 = property on="ConnectAll" class="Bool (strict)"("Disabled"=w427) -> ()  [unwired: 2 in, 2 out]
            n334 = property on="Set Output ON All" class="Bool (strict)"("Disabled"=w427) -> ()  [unwired: 2 in, 2 out]
            n335 = property on="AddChannel" class="Bool (strict)"("Disabled"=w427) -> ()  [unwired: 2 in, 2 out]
            n336 = property on="DisconnectChannel" class="Bool (strict)"("Disabled"=w427) -> ()  [unwired: 2 in, 2 out]
            n337 = property on="ReadFromFile" class="Bool (strict)"("Disabled"=w427) -> ()  [unwired: 2 in, 2 out]
            n338 = property on="ConnectChannel" class="Bool (strict)"("Disabled"=w427) -> ()  [unwired: 2 in, 2 out]
            n339 = property on="Quit" class="Bool (strict)"("Disabled"=w427) -> ()  [unwired: 2 in, 2 out]
            n340 = property on="DeleteChannel" class="Bool (strict)"("Disabled"=w427) -> ()  [unwired: 2 in, 2 out]
            n341 = property on="WriteToFile" class="Bool (strict)"("Disabled"=w427) -> ()  [unwired: 2 in, 2 out]
            n342 = property on="SetCurrentB" class="Bool (strict)"("Disabled"=w427) -> ()  [unwired: 2 in, 2 out]
            n343 = property on="SetOutputOnB" class="Bool (strict)"("Disabled"=w427) -> ()  [unwired: 2 in, 2 out]
            n344 = property on="SetVoltageB" class="Bool (strict)"("Disabled"=w427) -> ()  [unwired: 2 in, 2 out]
            n345 = property on="SetOutputOffB" class="Bool (strict)"("Disabled"=w427) -> ()  [unwired: 2 in, 2 out]
            n346 = property on="SetVoltageAll" class="Bool (strict)"("Disabled"=w427) -> ()  [unwired: 2 in, 2 out]
            n347 = property on="SetCurrentAll" class="Bool (strict)"("Disabled"=w427) -> ()  [unwired: 2 in, 2 out]
            n348 = property on="DisconnectAll" class="Bool (strict)"("Disabled"=w427) -> ()  [unwired: 2 in, 2 out]
          }
        }
        n349 = Merge Errors(w400) -> (w398:errorcluster)
      }
      event "ConnectAll": Value Change {
        n350 = event-data() -> ()  [unwired: 7 out]
        n351 = flat-sequence {
          tunnel: [w433] -> w430
          tunnel: [w442] -> w431
          tunnel: w430 -> [w442]
          frame #0 {
            w432 = u8 2 ("Disabled")
            n352 = property on="Quit" class="Bool (strict)"("Disabled"=w432) -> ()  [unwired: 2 in, 2 out]
            n353 = property on="ReadFromFile" class="Bool (strict)"("Disabled"=w432) -> ()  [unwired: 2 in, 2 out]
            n354 = property on="WriteToFile" class="Bool (strict)"("Disabled"=w432) -> ()  [unwired: 2 in, 2 out]
            n355 = property on="ConnectAll" class="Bool (strict)"("Disabled"=w432) -> ()  [unwired: 2 in, 2 out]
            n356 = property on="Set Output ON All" class="Bool (strict)"("Disabled"=w432) -> ()  [unwired: 2 in, 2 out]
            n357 = property on="SetOutputOffB" class="Bool (strict)"("Disabled"=w432) -> ()  [unwired: 2 in, 2 out]
            n358 = property on="AddChannel" class="Bool (strict)"("Disabled"=w432) -> ()  [unwired: 2 in, 2 out]
            n359 = property on="DisconnectChannel" class="Bool (strict)"("Disabled"=w432) -> ()  [unwired: 2 in, 2 out]
            n360 = property on="SetCurrentAll" class="Bool (strict)"("Disabled"=w432) -> ()  [unwired: 2 in, 2 out]
            n361 = property on="SetOutputOnB" class="Bool (strict)"("Disabled"=w432) -> ()  [unwired: 2 in, 2 out]
            n362 = property on="ConnectChannel" class="Bool (strict)"("Disabled"=w432) -> ()  [unwired: 2 in, 2 out]
            n363 = property on="DeleteChannel" class="Bool (strict)"("Disabled"=w432) -> ()  [unwired: 2 in, 2 out]
            n364 = property on="SetCurrentB" class="Bool (strict)"("Disabled"=w432) -> ()  [unwired: 2 in, 2 out]
            n365 = property on="SetVoltageB" class="Bool (strict)"("Disabled"=w432) -> ()  [unwired: 2 in, 2 out]
            n366 = property on="SetVoltageAll" class="Bool (strict)"("Disabled"=w432) -> ()  [unwired: 2 in, 2 out]
            n367 = property on="DisconnectAll" class="Bool (strict)"("Disabled"=w432) -> ()  [unwired: 2 in, 2 out]
          }
          frame #1 {
            n368 = local read "Measure_VI"() -> (w435:refnum<vi>[])
            n369 = Array Size(array=w435) -> (size(s)=w434:i32)
            n370 = for {
              N: w434 -> [_]
              tunnel: [w436] -> w433 mode=indexing
              i -> [w437]
              n371 = local read "Measure_VI"() -> (w440:refnum<vi>[])
              n372 = Index Array(array=w440, index=w437) -> (element=w439:refnum<vi>)
              n373 = invoke class="VI" method="Ctrl Val.Set"(reference=w439, "Control Name"="Connect", "Value"=TRUE ("OK Button")) -> (error out=w436:errorcluster)  [unwired: 2 in, 4 out]
            }
          }
          frame #2 {
            w443 = u8 0 ("Disabled")
            n374 = local write "ConnectAll"(FALSE ("ConnectChannel")) -> ()
            n375 = property on="Quit" class="Bool (strict)"("Disabled"=w443) -> ()  [unwired: 2 in, 2 out]
            n376 = property on="AddChannel" class="Bool (strict)"("Disabled"=w443) -> ()  [unwired: 2 in, 2 out]
            n377 = property on="DisconnectChannel" class="Bool (strict)"("Disabled"=w443) -> ()  [unwired: 2 in, 2 out]
            n378 = property on="ConnectAll" class="Bool (strict)"("Disabled"=w443) -> ()  [unwired: 2 in, 2 out]
            n379 = property on="Set Output ON All" class="Bool (strict)"("Disabled"=w443) -> ()  [unwired: 2 in, 2 out]
            n380 = property on="SetOutputOffB" class="Bool (strict)"("Disabled"=w443) -> ()  [unwired: 2 in, 2 out]
            n381 = property on="SetCurrentAll" class="Bool (strict)"("Disabled"=w443) -> ()  [unwired: 2 in, 2 out]
            n382 = property on="ConnectChannel" class="Bool (strict)"("Disabled"=w443) -> ()  [unwired: 2 in, 2 out]
            n383 = property on="SetVoltageAll" class="Bool (strict)"("Disabled"=w443) -> ()  [unwired: 2 in, 2 out]
            n384 = property on="SetOutputOnB" class="Bool (strict)"("Disabled"=w443) -> ()  [unwired: 2 in, 2 out]
            n385 = property on="DisconnectAll" class="Bool (strict)"("Disabled"=w443) -> ()  [unwired: 2 in, 2 out]
            n386 = property on="ReadFromFile" class="Bool (strict)"("Disabled"=w443) -> ()  [unwired: 2 in, 2 out]
            n387 = property on="WriteToFile" class="Bool (strict)"("Disabled"=w443) -> ()  [unwired: 2 in, 2 out]
            n388 = property on="SetCurrentB" class="Bool (strict)"("Disabled"=w443) -> ()  [unwired: 2 in, 2 out]
            n389 = property on="SetVoltageB" class="Bool (strict)"("Disabled"=w443) -> ()  [unwired: 2 in, 2 out]
            n390 = property on="DeleteChannel" class="Bool (strict)"("Disabled"=w443) -> ()  [unwired: 2 in, 2 out]
          }
        }
        n391 = Merge Errors(w431) -> (w429:errorcluster)
      }
      event "DisconnectAll": Value Change {
        n392 = event-data() -> ()  [unwired: 7 out]
        n393 = flat-sequence {
          tunnel: [w449] -> w447
          tunnel: [w458] -> w446
          tunnel: w447 -> [w458]
          frame #0 {
            w448 = u8 2 ("Disabled")
            n394 = property on="Quit" class="Bool (strict)"("Disabled"=w448) -> ()  [unwired: 2 in, 2 out]
            n395 = property on="ReadFromFile" class="Bool (strict)"("Disabled"=w448) -> ()  [unwired: 2 in, 2 out]
            n396 = property on="ConnectAll" class="Bool (strict)"("Disabled"=w448) -> ()  [unwired: 2 in, 2 out]
            n397 = property on="ConnectChannel" class="Bool (strict)"("Disabled"=w448) -> ()  [unwired: 2 in, 2 out]
            n398 = property on="AddChannel" class="Bool (strict)"("Disabled"=w448) -> ()  [unwired: 2 in, 2 out]
            n399 = property on="DisconnectChannel" class="Bool (strict)"("Disabled"=w448) -> ()  [unwired: 2 in, 2 out]
            n400 = property on="Set Output ON All" class="Bool (strict)"("Disabled"=w448) -> ()  [unwired: 2 in, 2 out]
            n401 = property on="WriteToFile" class="Bool (strict)"("Disabled"=w448) -> ()  [unwired: 2 in, 2 out]
            n402 = property on="SetOutputOffB" class="Bool (strict)"("Disabled"=w448) -> ()  [unwired: 2 in, 2 out]
            n403 = property on="SetCurrentAll" class="Bool (strict)"("Disabled"=w448) -> ()  [unwired: 2 in, 2 out]
            n404 = property on="SetOutputOnB" class="Bool (strict)"("Disabled"=w448) -> ()  [unwired: 2 in, 2 out]
            n405 = property on="DeleteChannel" class="Bool (strict)"("Disabled"=w448) -> ()  [unwired: 2 in, 2 out]
            n406 = property on="SetCurrentB" class="Bool (strict)"("Disabled"=w448) -> ()  [unwired: 2 in, 2 out]
            n407 = property on="SetVoltageB" class="Bool (strict)"("Disabled"=w448) -> ()  [unwired: 2 in, 2 out]
            n408 = property on="SetVoltageAll" class="Bool (strict)"("Disabled"=w448) -> ()  [unwired: 2 in, 2 out]
            n409 = property on="DisconnectAll" class="Bool (strict)"("Disabled"=w448) -> ()  [unwired: 2 in, 2 out]
          }
          frame #1 {
            n410 = local read "Measure_VI"() -> (w451:refnum<vi>[])
            n411 = Array Size(array=w451) -> (size(s)=w450:i32)
            n412 = for {
              N: w450 -> [_]
              tunnel: [w452] -> w449 mode=indexing
              i -> [w453]
              n413 = local read "Measure_VI"() -> (w456:refnum<vi>[])
              n414 = Index Array(array=w456, index=w453) -> (element=w455:refnum<vi>)
              n415 = invoke class="VI" method="Ctrl Val.Set"(reference=w455, "Control Name"="Connect", "Value"=FALSE ("OK Button")) -> (error out=w452:errorcluster)  [unwired: 2 in, 4 out]
            }
          }
          frame #2 {
            w459 = u8 0 ("Disabled")
            n416 = local write "DisconnectAll"(FALSE ("ConnectChannel")) -> ()
            n417 = property on="Quit" class="Bool (strict)"("Disabled"=w459) -> ()  [unwired: 2 in, 2 out]
            n418 = property on="ConnectAll" class="Bool (strict)"("Disabled"=w459) -> ()  [unwired: 2 in, 2 out]
            n419 = property on="ConnectChannel" class="Bool (strict)"("Disabled"=w459) -> ()  [unwired: 2 in, 2 out]
            n420 = property on="AddChannel" class="Bool (strict)"("Disabled"=w459) -> ()  [unwired: 2 in, 2 out]
            n421 = property on="DisconnectChannel" class="Bool (strict)"("Disabled"=w459) -> ()  [unwired: 2 in, 2 out]
            n422 = property on="ReadFromFile" class="Bool (strict)"("Disabled"=w459) -> ()  [unwired: 2 in, 2 out]
            n423 = property on="Set Output ON All" class="Bool (strict)"("Disabled"=w459) -> ()  [unwired: 2 in, 2 out]
            n424 = property on="WriteToFile" class="Bool (strict)"("Disabled"=w459) -> ()  [unwired: 2 in, 2 out]
            n425 = property on="SetOutputOnB" class="Bool (strict)"("Disabled"=w459) -> ()  [unwired: 2 in, 2 out]
            n426 = property on="SetCurrentB" class="Bool (strict)"("Disabled"=w459) -> ()  [unwired: 2 in, 2 out]
            n427 = property on="SetVoltageB" class="Bool (strict)"("Disabled"=w459) -> ()  [unwired: 2 in, 2 out]
            n428 = property on="SetVoltageAll" class="Bool (strict)"("Disabled"=w459) -> ()  [unwired: 2 in, 2 out]
            n429 = property on="DisconnectAll" class="Bool (strict)"("Disabled"=w459) -> ()  [unwired: 2 in, 2 out]
            n430 = property on="DeleteChannel" class="Bool (strict)"("Disabled"=w459) -> ()  [unwired: 2 in, 2 out]
            n431 = property on="SetOutputOffB" class="Bool (strict)"("Disabled"=w459) -> ()  [unwired: 2 in, 2 out]
            n432 = property on="SetCurrentAll" class="Bool (strict)"("Disabled"=w459) -> ()  [unwired: 2 in, 2 out]
          }
        }
        n433 = Merge Errors(w446) -> (w445:errorcluster)
      }
      event "SetVoltageB": Value Change {
        n434 = event-data() -> ()  [unwired: 7 out]
        n435 = local write "SetVoltageB"(FALSE ("ConnectChannel")) -> ()
        n436 = flat-sequence {
          tunnel: [w467] -> w463
          tunnel: [w476] -> w462
          tunnel: w463 -> [w476]
          frame #0 {
            w465 = u8 2 ("Disabled")
            n437 = property on="Quit" class="Bool (strict)"("Disabled"=w465) -> ()  [unwired: 2 in, 2 out]
            n438 = property on="AddChannel" class="Bool (strict)"("Disabled"=w465) -> ()  [unwired: 2 in, 2 out]
            n439 = property on="Set Output ON All" class="Bool (strict)"("Disabled"=w465) -> ()  [unwired: 2 in, 2 out]
            n440 = property on="ConnectAll" class="Bool (strict)"("Disabled"=w465) -> ()  [unwired: 2 in, 2 out]
            n441 = property on="DisconnectChannel" class="Bool (strict)"("Disabled"=w465) -> ()  [unwired: 2 in, 2 out]
            n442 = property on="ReadFromFile" class="Bool (strict)"("Disabled"=w465) -> ()  [unwired: 2 in, 2 out]
            n443 = property on="ConnectChannel" class="Bool (strict)"("Disabled"=w465) -> ()  [unwired: 2 in, 2 out]
            n444 = property on="DeleteChannel" class="Bool (strict)"("Disabled"=w465) -> ()  [unwired: 2 in, 2 out]
            n445 = property on="WriteToFile" class="Bool (strict)"("Disabled"=w465) -> ()  [unwired: 2 in, 2 out]
            n446 = property on="SetCurrentB" class="Bool (strict)"("Disabled"=w465) -> ()  [unwired: 2 in, 2 out]
            n447 = property on="SetOutputOnB" class="Bool (strict)"("Disabled"=w465) -> ()  [unwired: 2 in, 2 out]
            n448 = property on="SetVoltageB" class="Bool (strict)"("Disabled"=w465) -> ()  [unwired: 2 in, 2 out]
            n449 = property on="SetOutputOffB" class="Bool (strict)"("Disabled"=w465) -> ()  [unwired: 2 in, 2 out]
            n450 = property on="SetVoltageAll" class="Bool (strict)"("Disabled"=w465) -> ()  [unwired: 2 in, 2 out]
            n451 = property on="SetCurrentAll" class="Bool (strict)"("Disabled"=w465) -> ()  [unwired: 2 in, 2 out]
            n452 = property on="DisconnectAll" class="Bool (strict)"("Disabled"=w465) -> ()  [unwired: 2 in, 2 out]
          }
          frame #1 {
            n453 = property on="List of channels" class="MCListbox (strict)"() -> ("Value"=w466:i32)  [unwired: 2 in, 2 out]
            n454 = local read "Measure_VI"() -> (w474:refnum<vi>[])
            n455 = local read "SetVoltage"() -> (w472:dbl)
            n456 = Index Array(array=w474, index=w466) -> (element=w473:refnum<vi>)
            n457 = invoke class="VI" method="Ctrl Val.Set"(reference=w473, "Control Name"="SetVoltage", "Value"=w472) -> (reference out=w469:refnum<vi>, error out=w468:errorcluster)  [unwired: 2 in, 3 out]
            n458 = invoke class="VI" method="Ctrl Val.Set"(reference=w469, error in=w468, "Control Name"="NeedToSetVoltage", "Value"=TRUE ("ConnectChannel")) -> (error out=w467:errorcluster)  [unwired: 1 in, 4 out]
          }
          frame #2 {
            w477 = u8 0 ("Disabled")
            n459 = property on="Quit" class="Bool (strict)"("Disabled"=w477) -> ()  [unwired: 2 in, 2 out]
            n460 = property on="ConnectAll" class="Bool (strict)"("Disabled"=w477) -> ()  [unwired: 2 in, 2 out]
            n461 = property on="Set Output ON All" class="Bool (strict)"("Disabled"=w477) -> ()  [unwired: 2 in, 2 out]
            n462 = property on="AddChannel" class="Bool (strict)"("Disabled"=w477) -> ()  [unwired: 2 in, 2 out]
            n463 = property on="DisconnectChannel" class="Bool (strict)"("Disabled"=w477) -> ()  [unwired: 2 in, 2 out]
            n464 = property on="ReadFromFile" class="Bool (strict)"("Disabled"=w477) -> ()  [unwired: 2 in, 2 out]
            n465 = property on="ConnectChannel" class="Bool (strict)"("Disabled"=w477) -> ()  [unwired: 2 in, 2 out]
            n466 = property on="DeleteChannel" class="Bool (strict)"("Disabled"=w477) -> ()  [unwired: 2 in, 2 out]
            n467 = property on="SetVoltageAll" class="Bool (strict)"("Disabled"=w477) -> ()  [unwired: 2 in, 2 out]
            n468 = property on="SetCurrentAll" class="Bool (strict)"("Disabled"=w477) -> ()  [unwired: 2 in, 2 out]
            n469 = property on="DisconnectAll" class="Bool (strict)"("Disabled"=w477) -> ()  [unwired: 2 in, 2 out]
            n470 = property on="WriteToFile" class="Bool (strict)"("Disabled"=w477) -> ()  [unwired: 2 in, 2 out]
            n471 = property on="SetCurrentB" class="Bool (strict)"("Disabled"=w477) -> ()  [unwired: 2 in, 2 out]
            n472 = property on="SetOutputOnB" class="Bool (strict)"("Disabled"=w477) -> ()  [unwired: 2 in, 2 out]
            n473 = property on="SetVoltageB" class="Bool (strict)"("Disabled"=w477) -> ()  [unwired: 2 in, 2 out]
            n474 = property on="SetOutputOffB" class="Bool (strict)"("Disabled"=w477) -> ()  [unwired: 2 in, 2 out]
          }
        }
        n475 = Merge Errors(w462) -> (w461:errorcluster)
      }
      event "SetOutputOnB": Value Change {
        n476 = event-data() -> ()  [unwired: 2 out]
        n477 = property on="List of channels" class="MCListbox (strict)"() -> ("Value"=w481:i32)  [unwired: 2 in, 2 out]
        n478 = flat-sequence {
          tunnel: w481 -> [w483]
          tunnel: [w483] -> w480
          tunnel: w480 -> [w490]
          tunnel: [w485] -> w479
          tunnel: [w495] -> w478
          tunnel: w479 -> [w495]
          frame #0 {
            w482 = u8 2 ("Disabled")
            n479 = property on="ConnectAll" class="Bool (strict)"("Disabled"=w482) -> ()  [unwired: 2 in, 2 out]
            n480 = property on="Set Output ON All" class="Bool (strict)"("Disabled"=w482) -> ()  [unwired: 2 in, 2 out]
            n481 = property on="AddChannel" class="Bool (strict)"("Disabled"=w482) -> ()  [unwired: 2 in, 2 out]
            n482 = property on="DisconnectChannel" class="Bool (strict)"("Disabled"=w482) -> ()  [unwired: 2 in, 2 out]
            n483 = property on="ReadFromFile" class="Bool (strict)"("Disabled"=w482) -> ()  [unwired: 2 in, 2 out]
            n484 = property on="Quit" class="Bool (strict)"("Disabled"=w482) -> ()  [unwired: 2 in, 2 out]
            n485 = property on="ConnectChannel" class="Bool (strict)"("Disabled"=w482) -> ()  [unwired: 2 in, 2 out]
            n486 = property on="DeleteChannel" class="Bool (strict)"("Disabled"=w482) -> ()  [unwired: 2 in, 2 out]
            n487 = property on="WriteToFile" class="Bool (strict)"("Disabled"=w482) -> ()  [unwired: 2 in, 2 out]
            n488 = property on="SetCurrentB" class="Bool (strict)"("Disabled"=w482) -> ()  [unwired: 2 in, 2 out]
            n489 = property on="SetOutputOnB" class="Bool (strict)"("Disabled"=w482) -> ()  [unwired: 2 in, 2 out]
            n490 = property on="SetVoltageB" class="Bool (strict)"("Disabled"=w482) -> ()  [unwired: 2 in, 2 out]
            n491 = property on="SetOutputOffB" class="Bool (strict)"("Disabled"=w482) -> ()  [unwired: 2 in, 2 out]
            n492 = property on="SetVoltageAll" class="Bool (strict)"("Disabled"=w482) -> ()  [unwired: 2 in, 2 out]
            n493 = property on="SetCurrentAll" class="Bool (strict)"("Disabled"=w482) -> ()  [unwired: 2 in, 2 out]
            n494 = property on="DisconnectAll" class="Bool (strict)"("Disabled"=w482) -> ()  [unwired: 2 in, 2 out]
          }
          frame #1 {
            n495 = local write "SetOutputOnB"(FALSE ("ConnectChannel")) -> ()
            n496 = local read "Measure_VI"() -> (w493:refnum<vi>[])
            n497 = Index Array(array=w493, index=w490) -> (element=w492:refnum<vi>)
            n498 = invoke class="VI" method="Ctrl Val.Set"(reference=w492, "Control Name"="SetOutput", "Value"=TRUE ("ConnectChannel")) -> (reference out=w487:refnum<vi>, error out=w486:errorcluster)  [unwired: 2 in, 3 out]
            n499 = invoke class="VI" method="Ctrl Val.Set"(reference=w487, error in=w486, "Control Name"="NeedToSetOutput", "Value"=TRUE ("ConnectChannel")) -> (error out=w485:errorcluster)  [unwired: 1 in, 4 out]
          }
          frame #2 {
            w496 = u8 0 ("Disabled")
            n500 = property on="ConnectAll" class="Bool (strict)"("Disabled"=w496) -> ()  [unwired: 2 in, 2 out]
            n501 = property on="Set Output ON All" class="Bool (strict)"("Disabled"=w496) -> ()  [unwired: 2 in, 2 out]
            n502 = property on="AddChannel" class="Bool (strict)"("Disabled"=w496) -> ()  [unwired: 2 in, 2 out]
            n503 = property on="DisconnectChannel" class="Bool (strict)"("Disabled"=w496) -> ()  [unwired: 2 in, 2 out]
            n504 = property on="ReadFromFile" class="Bool (strict)"("Disabled"=w496) -> ()  [unwired: 2 in, 2 out]
            n505 = property on="ConnectChannel" class="Bool (strict)"("Disabled"=w496) -> ()  [unwired: 2 in, 2 out]
            n506 = property on="Quit" class="Bool (strict)"("Disabled"=w496) -> ()  [unwired: 2 in, 2 out]
            n507 = property on="DeleteChannel" class="Bool (strict)"("Disabled"=w496) -> ()  [unwired: 2 in, 2 out]
            n508 = property on="SetOutputOffB" class="Bool (strict)"("Disabled"=w496) -> ()  [unwired: 2 in, 2 out]
            n509 = property on="SetVoltageAll" class="Bool (strict)"("Disabled"=w496) -> ()  [unwired: 2 in, 2 out]
            n510 = property on="SetCurrentAll" class="Bool (strict)"("Disabled"=w496) -> ()  [unwired: 2 in, 2 out]
            n511 = property on="DisconnectAll" class="Bool (strict)"("Disabled"=w496) -> ()  [unwired: 2 in, 2 out]
            n512 = property on="WriteToFile" class="Bool (strict)"("Disabled"=w496) -> ()  [unwired: 2 in, 2 out]
            n513 = property on="SetCurrentB" class="Bool (strict)"("Disabled"=w496) -> ()  [unwired: 2 in, 2 out]
            n514 = property on="SetOutputOnB" class="Bool (strict)"("Disabled"=w496) -> ()  [unwired: 2 in, 2 out]
            n515 = property on="SetVoltageB" class="Bool (strict)"("Disabled"=w496) -> ()  [unwired: 2 in, 2 out]
          }
        }
      }
      event "Set Output ON All": Value Change {
        n516 = event-data() -> ("NewVal"=w497:bool)  [unwired: 1 out]
        n517 = flat-sequence {
          tunnel: [w502] -> w498
          tunnel: w497 -> [w502]
          tunnel: [w507] -> w500
          tunnel: w498 -> [w504]
          tunnel: [w518] -> w501
          tunnel: w500 -> [w518]
          frame #0 {
            w503 = u8 2 ("Disabled")
            n518 = property on="Quit" class="Bool (strict)"("Disabled"=w503) -> ()  [unwired: 2 in, 2 out]
            n519 = property on="AddChannel" class="Bool (strict)"("Disabled"=w503) -> ()  [unwired: 2 in, 2 out]
            n520 = property on="DisconnectChannel" class="Bool (strict)"("Disabled"=w503) -> ()  [unwired: 2 in, 2 out]
            n521 = property on="ConnectAll" class="Bool (strict)"("Disabled"=w503) -> ()  [unwired: 2 in, 2 out]
            n522 = property on="ReadFromFile" class="Bool (strict)"("Disabled"=w503) -> ()  [unwired: 2 in, 2 out]
            n523 = property on="ConnectChannel" class="Bool (strict)"("Disabled"=w503) -> ()  [unwired: 2 in, 2 out]
            n524 = property on="DeleteChannel" class="Bool (strict)"("Disabled"=w503) -> ()  [unwired: 2 in, 2 out]
            n525 = property on="WriteToFile" class="Bool (strict)"("Disabled"=w503) -> ()  [unwired: 2 in, 2 out]
            n526 = property on="SetCurrentB" class="Bool (strict)"("Disabled"=w503) -> ()  [unwired: 2 in, 2 out]
            n527 = property on="SetOutputOnB" class="Bool (strict)"("Disabled"=w503) -> ()  [unwired: 2 in, 2 out]
            n528 = property on="SetVoltageB" class="Bool (strict)"("Disabled"=w503) -> ()  [unwired: 2 in, 2 out]
            n529 = property on="SetOutputOffB" class="Bool (strict)"("Disabled"=w503) -> ()  [unwired: 2 in, 2 out]
            n530 = property on="SetVoltageAll" class="Bool (strict)"("Disabled"=w503) -> ()  [unwired: 2 in, 2 out]
            n531 = property on="SetCurrentAll" class="Bool (strict)"("Disabled"=w503) -> ()  [unwired: 2 in, 2 out]
            n532 = property on="DisconnectAll" class="Bool (strict)"("Disabled"=w503) -> ()  [unwired: 2 in, 2 out]
          }
          frame #1 {
            n533 = local read "Measure_VI"() -> (w506:refnum<vi>[])
            n534 = Array Size(array=w506) -> (size(s)=w505:i32)
            n535 = for {
              N: w505 -> [_]
              tunnel: [w509] -> w507 mode=indexing
              tunnel: w504 -> [w508]
              i -> [w511]
              n536 = local read "Measure_VI"() -> (w516:refnum<vi>[])
              n537 = Index Array(array=w516, index=w511) -> (element=w515:refnum<vi>)
              n538 = invoke class="VI" method="Ctrl Val.Set"(reference=w515, "Control Name"="SetOutput", "Value"=w508) -> (reference out=w512:refnum<vi>, error out=w510:errorcluster)  [unwired: 2 in, 3 out]
              n539 = invoke class="VI" method="Ctrl Val.Set"(reference=w512, error in=w510, "Control Name"="NeedToSetOutput", "Value"=TRUE ("ConnectChannel")) -> (error out=w509:errorcluster)  [unwired: 1 in, 4 out]
            }
          }
          frame #2 {
            w519 = u8 0 ("Disabled")
            n540 = disable-structure shown="Disabled" {
              frame Disabled {
                n541 = local write "Set Output ON All"(FALSE ("ConnectChannel")) -> ()
              }
              frame Enabled {
              }
            }
            n542 = property on="Quit" class="Bool (strict)"("Disabled"=w519) -> ()  [unwired: 2 in, 2 out]
            n543 = property on="ConnectAll" class="Bool (strict)"("Disabled"=w519) -> ()  [unwired: 2 in, 2 out]
            n544 = property on="Set Output ON All" class="Bool (strict)"("Disabled"=w519) -> ()  [unwired: 2 in, 2 out]
            n545 = property on="AddChannel" class="Bool (strict)"("Disabled"=w519) -> ()  [unwired: 2 in, 2 out]
            n546 = property on="DisconnectChannel" class="Bool (strict)"("Disabled"=w519) -> ()  [unwired: 2 in, 2 out]
            n547 = property on="ReadFromFile" class="Bool (strict)"("Disabled"=w519) -> ()  [unwired: 2 in, 2 out]
            n548 = property on="ConnectChannel" class="Bool (strict)"("Disabled"=w519) -> ()  [unwired: 2 in, 2 out]
            n549 = property on="DeleteChannel" class="Bool (strict)"("Disabled"=w519) -> ()  [unwired: 2 in, 2 out]
            n550 = property on="SetVoltageB" class="Bool (strict)"("Disabled"=w519) -> ()  [unwired: 2 in, 2 out]
            n551 = property on="SetOutputOffB" class="Bool (strict)"("Disabled"=w519) -> ()  [unwired: 2 in, 2 out]
            n552 = property on="SetVoltageAll" class="Bool (strict)"("Disabled"=w519) -> ()  [unwired: 2 in, 2 out]
            n553 = property on="SetCurrentAll" class="Bool (strict)"("Disabled"=w519) -> ()  [unwired: 2 in, 2 out]
            n554 = property on="DisconnectAll" class="Bool (strict)"("Disabled"=w519) -> ()  [unwired: 2 in, 2 out]
            n555 = property on="WriteToFile" class="Bool (strict)"("Disabled"=w519) -> ()  [unwired: 2 in, 2 out]
            n556 = property on="SetCurrentB" class="Bool (strict)"("Disabled"=w519) -> ()  [unwired: 2 in, 2 out]
            n557 = property on="SetOutputOnB" class="Bool (strict)"("Disabled"=w519) -> ()  [unwired: 2 in, 2 out]
          }
        }
        n558 = Merge Errors(w501) -> (w499:errorcluster)
      }
      event "SetOutputOffB": Value Change {
        n559 = event-data() -> ()  [unwired: 7 out]
        n560 = local write "SetOutputOffB"(FALSE ("ConnectChannel")) -> ()
        n561 = property on="List of channels" class="MCListbox (strict)"() -> ("Value"=w525:i32)  [unwired: 2 in, 2 out]
        n562 = flat-sequence {
          tunnel: w525 -> [w527]
          tunnel: [w527] -> w524
          tunnel: w524 -> [w534]
          tunnel: [w528] -> w521
          tunnel: [w538] -> w522
          tunnel: w521 -> [w538]
          frame #0 {
            w526 = u8 2 ("Disabled")
            n563 = property on="ConnectAll" class="Bool (strict)"("Disabled"=w526) -> ()  [unwired: 2 in, 2 out]
            n564 = property on="Set Output ON All" class="Bool (strict)"("Disabled"=w526) -> ()  [unwired: 2 in, 2 out]
            n565 = property on="AddChannel" class="Bool (strict)"("Disabled"=w526) -> ()  [unwired: 2 in, 2 out]
            n566 = property on="DisconnectChannel" class="Bool (strict)"("Disabled"=w526) -> ()  [unwired: 2 in, 2 out]
            n567 = property on="ReadFromFile" class="Bool (strict)"("Disabled"=w526) -> ()  [unwired: 2 in, 2 out]
            n568 = property on="Quit" class="Bool (strict)"("Disabled"=w526) -> ()  [unwired: 2 in, 2 out]
            n569 = property on="ConnectChannel" class="Bool (strict)"("Disabled"=w526) -> ()  [unwired: 2 in, 2 out]
            n570 = property on="DeleteChannel" class="Bool (strict)"("Disabled"=w526) -> ()  [unwired: 2 in, 2 out]
            n571 = property on="WriteToFile" class="Bool (strict)"("Disabled"=w526) -> ()  [unwired: 2 in, 2 out]
            n572 = property on="SetCurrentB" class="Bool (strict)"("Disabled"=w526) -> ()  [unwired: 2 in, 2 out]
            n573 = property on="SetOutputOnB" class="Bool (strict)"("Disabled"=w526) -> ()  [unwired: 2 in, 2 out]
            n574 = property on="SetVoltageB" class="Bool (strict)"("Disabled"=w526) -> ()  [unwired: 2 in, 2 out]
            n575 = property on="SetOutputOffB" class="Bool (strict)"("Disabled"=w526) -> ()  [unwired: 2 in, 2 out]
            n576 = property on="SetVoltageAll" class="Bool (strict)"("Disabled"=w526) -> ()  [unwired: 2 in, 2 out]
            n577 = property on="SetCurrentAll" class="Bool (strict)"("Disabled"=w526) -> ()  [unwired: 2 in, 2 out]
            n578 = property on="DisconnectAll" class="Bool (strict)"("Disabled"=w526) -> ()  [unwired: 2 in, 2 out]
          }
          frame #1 {
            n579 = local read "Measure_VI"() -> (w536:refnum<vi>[])
            n580 = Index Array(array=w536, index=w534) -> (element=w535:refnum<vi>)
            n581 = invoke class="VI" method="Ctrl Val.Set"(reference=w535, "Control Name"="SetOutput", "Value"=FALSE ("ConnectChannel")) -> (reference out=w531:refnum<vi>, error out=w529:errorcluster)  [unwired: 2 in, 3 out]
            n582 = invoke class="VI" method="Ctrl Val.Set"(reference=w531, error in=w529, "Control Name"="NeedToSetOutput", "Value"=TRUE ("ConnectChannel")) -> (error out=w528:errorcluster)  [unwired: 1 in, 4 out]
          }
          frame #2 {
            w539 = u8 0 ("Disabled")
            n583 = property on="ConnectAll" class="Bool (strict)"("Disabled"=w539) -> ()  [unwired: 2 in, 2 out]
            n584 = property on="Set Output ON All" class="Bool (strict)"("Disabled"=w539) -> ()  [unwired: 2 in, 2 out]
            n585 = property on="AddChannel" class="Bool (strict)"("Disabled"=w539) -> ()  [unwired: 2 in, 2 out]
            n586 = property on="DisconnectChannel" class="Bool (strict)"("Disabled"=w539) -> ()  [unwired: 2 in, 2 out]
            n587 = property on="ReadFromFile" class="Bool (strict)"("Disabled"=w539) -> ()  [unwired: 2 in, 2 out]
            n588 = property on="ConnectChannel" class="Bool (strict)"("Disabled"=w539) -> ()  [unwired: 2 in, 2 out]
            n589 = property on="Quit" class="Bool (strict)"("Disabled"=w539) -> ()  [unwired: 2 in, 2 out]
            n590 = property on="DeleteChannel" class="Bool (strict)"("Disabled"=w539) -> ()  [unwired: 2 in, 2 out]
            n591 = property on="SetOutputOffB" class="Bool (strict)"("Disabled"=w539) -> ()  [unwired: 2 in, 2 out]
            n592 = property on="SetVoltageAll" class="Bool (strict)"("Disabled"=w539) -> ()  [unwired: 2 in, 2 out]
            n593 = property on="SetCurrentAll" class="Bool (strict)"("Disabled"=w539) -> ()  [unwired: 2 in, 2 out]
            n594 = property on="DisconnectAll" class="Bool (strict)"("Disabled"=w539) -> ()  [unwired: 2 in, 2 out]
            n595 = property on="WriteToFile" class="Bool (strict)"("Disabled"=w539) -> ()  [unwired: 2 in, 2 out]
            n596 = property on="SetCurrentB" class="Bool (strict)"("Disabled"=w539) -> ()  [unwired: 2 in, 2 out]
            n597 = property on="SetOutputOnB" class="Bool (strict)"("Disabled"=w539) -> ()  [unwired: 2 in, 2 out]
            n598 = property on="SetVoltageB" class="Bool (strict)"("Disabled"=w539) -> ()  [unwired: 2 in, 2 out]
          }
        }
      }
      event "WriteToFile": Value Change {
        n599 = event-data() -> ()  [unwired: 7 out]
        n600 = local read "ADRESS"() -> (w544:string[])
        n601 = Array Size(array=w544) -> (size(s)=w543:i32)
        n602 = flat-sequence {
          tunnel: w543 -> [w553]
          tunnel: [w545] -> w541
          tunnel: [w586] -> w542
          tunnel: w541 -> [w586]
          frame #0 {
            n603 = Number To Decimal String(number=w553) -> (decimal integer string=w548:string)  [unwired: 1 out]
            n604 = Write to Text File(text=w548) -> (refnum out=w547:refnum<file>, cancelled=w546:bool, error out=w549:errorcluster)  [unwired: 1 in, 2 out]
            n605 = Write to Text File(file (use dialog)=w547, text="\nИМЯ  АДРЕС  ТОК  НАПРЯЖЕНИЕ", error in=w549) -> (refnum out=w550:refnum<file>, error out=w551:errorcluster)  [unwired: 2 out]
            n606 = for {
              N: w553 -> [_]
              tunnel: w546 -> [w563]
              tunnel: w551 -> [w558]
              tunnel: w550 -> [w565]
              tunnel: [w556] -> w545 mode=indexing
              i -> [w564]
              w569 = "" ("Control Name")
              w575 = "\t"
              n607 = local read "Measure_VI"() -> (w573:refnum<vi>[])
              n608 = Index Array(array=w573, index=w564) -> (element=w572:refnum<vi>)
              n609 = invoke class="VI" method="Ctrl Val.Get"(reference=w572, "Control Name"="SetVoltageStr") -> (reference out=w567:refnum<vi>, error out=w560:errorcluster, "Get Control Value Variant"=w574:variant)  [unwired: 2 in, 1 out]
              n610 = invoke class="VI" method="Ctrl Val.Get"(reference=w567, error in=w560, "Control Name"="SetCurrentStr") -> (error out=w559:errorcluster, "Get Control Value Variant"=w570:variant)  [unwired: 1 in, 2 out]
              n611 = local read "ADRESS"() -> (w580:string[])
              n612 = local read "NAME"() -> (w578:string[])
              n613 = Index Array(array=w578, index=w564) -> (element=w576:string)
              n614 = Index Array(array=w580, index=w564) -> (element=w579:string)
              n615 = Variant To Data(type=w569, Variant=w570) -> (data=w554:string, error out=w562:errorcluster)  [unwired: 1 in]
              n616 = Variant To Data(type=w569, Variant=w574) -> (data=w555:string, error out=w561:errorcluster)  [unwired: 1 in]
              n617 = Merge Errors(w559, w562, w561, w558) -> (w557:errorcluster)
              n618 = Concatenate Strings("\r\n", w576, w575, w579, w575, w554, w575, w555) -> (w566:string)
              n619 = case shown="False" w563 {
                tunnel: w565 -> [w583 _]
                tunnel: w566 -> [w584 _]
                tunnel: w557 -> [w582 w585]
                tunnel: [w581 w585] -> w556
                frame False {
                  n620 = Write to Text File(file (use dialog)=w583, text=w584, error in=w582) -> (error out=w581:errorcluster)  [unwired: 3 out]
                }
                frame True {
                }
              }
            }
          }
          frame #1 {
            n621 = local write "WriteToFile"(FALSE ("ConnectChannel")) -> ()
          }
        }
        n622 = Merge Errors(w542) -> (w540:errorcluster)
      }
      event "ReadFromFile": Value Change {
        n623 = event-data() -> ()  [unwired: 2 out]
        n624 = Read from Text File(count=100) -> (text=w594:string[], cancelled=w593:bool, error out=w592:errorcluster)  [unwired: 1 in, 3 out]
        n625 = local read "ReadFromFile"() -> (w590:bool)
        n626 = Not(x=w593) -> (.not. x?=w589:bool)
        n627 = And(x=w590, y=w589) -> (x .and. y?=w588:bool)
        n628 = case shown="True" w588 {
          tunnel: w594 -> [_ w598]
          tunnel: w592 -> [w596 w600]
          tunnel: [w596 w599] -> w591
          frame False {
            n629 = local write "ReadFromFile"(FALSE ("ConnectChannel")) -> ()
          }
          frame True {
            n630 = flat-sequence {
              tunnel: w600 -> [w607]
              tunnel: [w606] -> w602
              tunnel: w602 -> [w621]
              tunnel: [w621] -> w601
              tunnel: w601 -> [_]
              tunnel: [w630] -> w604
              tunnel: w598 -> [w632]
              tunnel: w604 -> [w666]
              tunnel: [w666] -> w603
              frame #0 {
                w605 = u8 2 ("Disabled")
                n631 = disable-structure shown="Enabled" {
                  disable-tunnel: w607 -> [w610 w619]
                  disable-tunnel: [w609 w619] -> w606
                  frame Disabled {
                    n632 = local read "Measure_VI"() -> (w611:refnum<vi>[])
                    n633 = Array Size(array=w611) -> (size(s)=w608:i32)
                    n634 = for {
                      N: w608 -> [_]
                      tunnel: w611 -> [w615]
                      tunnel: w610 -> [w613]
                      tunnel: [w612] -> w609 mode=indexing
                      i -> [w616]
                      n635 = Index Array(array=w615, index=w616) -> (element=w614:refnum<vi>)
                      n636 = invoke class="VI" method="Ctrl Val.Set"(reference=w614, error in=w613, "Control Name"="Connect", "Value"=FALSE) -> (error out=w612:errorcluster)  [unwired: 1 in, 4 out]
                    }
                  }
                  frame Enabled {
                  }
                }
                n637 = property on="Set Output ON All" class="Bool (strict)"("Disabled"=w605) -> ()  [unwired: 2 in, 2 out]
                n638 = property on="ConnectAll" class="Bool (strict)"("Disabled"=w605) -> ()  [unwired: 2 in, 2 out]
                n639 = property on="ReadFromFile" class="Bool (strict)"("Disabled"=w605) -> ()  [unwired: 2 in, 2 out]
                n640 = property on="ConnectChannel" class="Bool (strict)"("Disabled"=w605) -> ()  [unwired: 2 in, 2 out]
                n641 = property on="DisconnectChannel" class="Bool (strict)"("Disabled"=w605) -> ()  [unwired: 2 in, 2 out]
                n642 = property on="WriteToFile" class="Bool (strict)"("Disabled"=w605) -> ()  [unwired: 2 in, 2 out]
                n643 = property on="AddChannel" class="Bool (strict)"("Disabled"=w605) -> ()  [unwired: 2 in, 2 out]
                n644 = property on="SetOutputOnB" class="Bool (strict)"("Disabled"=w605) -> ()  [unwired: 2 in, 2 out]
                n645 = property on="Quit" class="Bool (strict)"("Disabled"=w605) -> ()  [unwired: 2 in, 2 out]
                n646 = property on="DeleteChannel" class="Bool (strict)"("Disabled"=w605) -> ()  [unwired: 2 in, 2 out]
                n647 = property on="SetCurrentB" class="Bool (strict)"("Disabled"=w605) -> ()  [unwired: 2 in, 2 out]
                n648 = property on="SetOutputOffB" class="Bool (strict)"("Disabled"=w605) -> ()  [unwired: 2 in, 2 out]
                n649 = property on="SetCurrentAll" class="Bool (strict)"("Disabled"=w605) -> ()  [unwired: 2 in, 2 out]
                n650 = property on="SetVoltageB" class="Bool (strict)"("Disabled"=w605) -> ()  [unwired: 2 in, 2 out]
                n651 = property on="SetVoltageAll" class="Bool (strict)"("Disabled"=w605) -> ()  [unwired: 2 in, 2 out]
                n652 = property on="DisconnectAll" class="Bool (strict)"("Disabled"=w605) -> ()  [unwired: 2 in, 2 out]
              }
              frame #1 {
                n653 = Wait (ms)(milliseconds to wait=u32 1000) -> ()  [unwired: 1 out]
              }
              frame #2 {
                n654 = local read "Measure_VI"() -> (w624:refnum<vi>[])
                n655 = Wait (ms)(milliseconds to wait=u32 250) -> ()  [unwired: 1 out]
                n656 = Array Size(array=w624) -> (size(s)=w623:i32)
                n657 = for {
                  N: w623 -> [_]
                  tunnel: w624 -> [w626]
                  i -> [w627]
                  n658 = Index Array(array=w626, index=w627) -> (element=w625:refnum<vi>)
                  n659 = invoke class="VI" method="Abort VI"(reference=w625) -> ()  [unwired: 2 in, 3 out]
                }
              }
              frame #3 {
                w629 = string[] [] ("GlobalInAdress")
                n660 = local write "NAME"(w629) -> ()
                n661 = local write "ADRESS"(w629) -> ()
                n662 = local write "Measure_VI"(refnum<vi>[] []) -> ()
              }
              frame #4 {
                n663 = Index Array(array=w632, index=0) -> (element=w635:string)
                n664 = Decimal String To Number(string=w635) -> (number=w633:i32)  [unwired: 3 out]
                n665 = for {
                  N: w633 -> [_]
                  tunnel: w632 -> [w660]
                  tunnel: [w638] -> w631 mode=indexing
                  i -> [w663]
                  n666 = Add(x=2, y=w663) -> (x+y=w662:i32)
                  n667 = Index Array(array=w660, index=w662) -> (element=w659:string)
                  n668 = Spreadsheet String To Array(format string="%s", spreadsheet string=w659, array type (2D Dbl)=string[] [] ("GlobalInAdress")) -> (array=w650:string[])  [unwired: 1 out]
                  n669 = Index Array(array=w650, index=2) -> (element=w636:string)
                  n670 = Index Array(array=w650, index=0) -> (element=w654:string)
                  n671 = Index Array(array=w650, index=1) -> (element=w655:string)
                  n672 = Index Array(array=w650, index=3) -> (element=w637:string)
                  n673 = local read "Measure_VI"() -> (w647:refnum<vi>[])
                  n674 = local read "ADRESS"() -> (w648:string[])
                  n675 = Scan From String(input string=w636, default 1=0.0 ("default value 1")) -> (output 1=w643:dbl)  [unwired: 3 in, 3 out]
                  n676 = Scan From String(input string=w637, default 1=0.0 ("default value 1")) -> (output 1=w645:dbl)  [unwired: 3 in, 3 out]
                  n677 = local read "NAME"() -> (w649:string[])
                  n678 = call "AddChannel.vi"("VIRef"=w647, "Name"=w654, "SetCurrent"=w643, "ADRESS"=w648, "NAME"=w649, "Address"=w655, "SetVoltage"=w645) -> ("NAMEOut"=w642:string[], "error out"=w639:errorcluster, "ADRESSOut"=w640:string[], "VIRefOut"=w641:refnum<vi>[])  [unwired: 1 in, 4 out]
                  n679 = local write "NAME"(w642) -> ()
                  n680 = flat-sequence {
                    tunnel: w639 -> [w665]
                    tunnel: [w665] -> w638
                    frame #0 {
                      n681 = Wait (ms)(milliseconds to wait=u32 50) -> ()  [unwired: 1 out]
                    }
                  }
                  n682 = local write "ADRESS"(w640) -> ()
                  n683 = local write "Measure_VI"(w641) -> ()
                }
                n684 = Merge Errors(w631) -> (w630:errorcluster)
              }
              frame #5 {
                w667 = u8 0 ("Disabled")
                n685 = local write "ReadFromFile"(FALSE ("ConnectChannel")) -> ()
                n686 = property on="ConnectAll" class="Bool (strict)"("Disabled"=w667) -> ()  [unwired: 2 in, 2 out]
                n687 = property on="Set Output ON All" class="Bool (strict)"("Disabled"=w667) -> ()  [unwired: 2 in, 2 out]
                n688 = property on="AddChannel" class="Bool (strict)"("Disabled"=w667) -> ()  [unwired: 2 in, 2 out]
                n689 = property on="DisconnectChannel" class="Bool (strict)"("Disabled"=w667) -> ()  [unwired: 2 in, 2 out]
                n690 = property on="ReadFromFile" class="Bool (strict)"("Disabled"=w667) -> ()  [unwired: 2 in, 2 out]
                n691 = property on="ConnectChannel" class="Bool (strict)"("Disabled"=w667) -> ()  [unwired: 2 in, 2 out]
                n692 = property on="DeleteChannel" class="Bool (strict)"("Disabled"=w667) -> ()  [unwired: 2 in, 2 out]
                n693 = property on="WriteToFile" class="Bool (strict)"("Disabled"=w667) -> ()  [unwired: 2 in, 2 out]
                n694 = property on="SetCurrentB" class="Bool (strict)"("Disabled"=w667) -> ()  [unwired: 2 in, 2 out]
                n695 = property on="Quit" class="Bool (strict)"("Disabled"=w667) -> ()  [unwired: 2 in, 2 out]
                n696 = property on="SetOutputOnB" class="Bool (strict)"("Disabled"=w667) -> ()  [unwired: 2 in, 2 out]
                n697 = property on="SetVoltageB" class="Bool (strict)"("Disabled"=w667) -> ()  [unwired: 2 in, 2 out]
                n698 = property on="SetOutputOffB" class="Bool (strict)"("Disabled"=w667) -> ()  [unwired: 2 in, 2 out]
                n699 = property on="SetVoltageAll" class="Bool (strict)"("Disabled"=w667) -> ()  [unwired: 2 in, 2 out]
                n700 = property on="SetCurrentAll" class="Bool (strict)"("Disabled"=w667) -> ()  [unwired: 2 in, 2 out]
                n701 = property on="DisconnectAll" class="Bool (strict)"("Disabled"=w667) -> ()  [unwired: 2 in, 2 out]
              }
            }
            n702 = Merge Errors(w603) -> (w599:errorcluster)
          }
        }
      }
      event "SetCurrentB": Value Change {
        n703 = event-data() -> ()  [unwired: 7 out]
        n704 = local write "SetCurrentB"(FALSE ("ConnectChannel")) -> ()
        n705 = property on="List of channels" class="MCListbox (strict)"() -> (error out=w671:errorcluster, "Value"=w675:i32)  [unwired: 2 in, 1 out]
        n706 = flat-sequence {
          tunnel: w675 -> [w678]
          tunnel: [w678] -> w674
          tunnel: [w676] -> w672
          tunnel: w671 -> [w676]
          tunnel: w674 -> [w680]
          tunnel: w672 -> [w679]
          tunnel: [w681] -> w670
          tunnel: [w690] -> w669
          tunnel: w670 -> [w690]
          frame #0 {
            w677 = u8 2 ("Disabled")
            n707 = property on="AddChannel" class="Bool (strict)"("Disabled"=w677) -> ()  [unwired: 2 in, 2 out]
            n708 = property on="Set Output ON All" class="Bool (strict)"("Disabled"=w677) -> ()  [unwired: 2 in, 2 out]
            n709 = property on="ConnectAll" class="Bool (strict)"("Disabled"=w677) -> ()  [unwired: 2 in, 2 out]
            n710 = property on="DisconnectChannel" class="Bool (strict)"("Disabled"=w677) -> ()  [unwired: 2 in, 2 out]
            n711 = property on="ReadFromFile" class="Bool (strict)"("Disabled"=w677) -> ()  [unwired: 2 in, 2 out]
            n712 = property on="Quit" class="Bool (strict)"("Disabled"=w677) -> ()  [unwired: 2 in, 2 out]
            n713 = property on="ConnectChannel" class="Bool (strict)"("Disabled"=w677) -> ()  [unwired: 2 in, 2 out]
            n714 = property on="DeleteChannel" class="Bool (strict)"("Disabled"=w677) -> ()  [unwired: 2 in, 2 out]
            n715 = property on="WriteToFile" class="Bool (strict)"("Disabled"=w677) -> ()  [unwired: 2 in, 2 out]
            n716 = property on="SetCurrentB" class="Bool (strict)"("Disabled"=w677) -> ()  [unwired: 2 in, 2 out]
            n717 = property on="SetOutputOnB" class="Bool (strict)"("Disabled"=w677) -> ()  [unwired: 2 in, 2 out]
            n718 = property on="SetVoltageB" class="Bool (strict)"("Disabled"=w677) -> ()  [unwired: 2 in, 2 out]
            n719 = property on="SetOutputOffB" class="Bool (strict)"("Disabled"=w677) -> ()  [unwired: 2 in, 2 out]
            n720 = property on="SetVoltageAll" class="Bool (strict)"("Disabled"=w677) -> ()  [unwired: 2 in, 2 out]
            n721 = property on="SetCurrentAll" class="Bool (strict)"("Disabled"=w677) -> ()  [unwired: 2 in, 2 out]
            n722 = property on="DisconnectAll" class="Bool (strict)"("Disabled"=w677) -> ()  [unwired: 2 in, 2 out]
          }
          frame #1 {
            n723 = local read "Measure_VI"() -> (w688:refnum<vi>[])
            n724 = local read "SetCurrent"() -> (w686:dbl)
            n725 = Index Array(array=w688, index=w680) -> (element=w687:refnum<vi>)
            n726 = invoke class="VI" method="Ctrl Val.Set"(reference=w687, error in=w679, "Control Name"="SetCurrent", "Value"=w686) -> (reference out=w683:refnum<vi>, error out=w682:errorcluster)  [unwired: 1 in, 3 out]
            n727 = invoke class="VI" method="Ctrl Val.Set"(reference=w683, error in=w682, "Control Name"="NeedToSetCurrent", "Value"=TRUE ("ConnectChannel")) -> (error out=w681:errorcluster)  [unwired: 1 in, 4 out]
          }
          frame #2 {
            w691 = u8 0 ("Disabled")
            n728 = property on="AddChannel" class="Bool (strict)"("Disabled"=w691) -> ()  [unwired: 2 in, 2 out]
            n729 = property on="Set Output ON All" class="Bool (strict)"("Disabled"=w691) -> ()  [unwired: 2 in, 2 out]
            n730 = property on="DisconnectChannel" class="Bool (strict)"("Disabled"=w691) -> ()  [unwired: 2 in, 2 out]
            n731 = property on="ConnectAll" class="Bool (strict)"("Disabled"=w691) -> ()  [unwired: 2 in, 2 out]
            n732 = property on="ReadFromFile" class="Bool (strict)"("Disabled"=w691) -> ()  [unwired: 2 in, 2 out]
            n733 = property on="ConnectChannel" class="Bool (strict)"("Disabled"=w691) -> ()  [unwired: 2 in, 2 out]
            n734 = property on="DeleteChannel" class="Bool (strict)"("Disabled"=w691) -> ()  [unwired: 2 in, 2 out]
            n735 = property on="Quit" class="Bool (strict)"("Disabled"=w691) -> ()  [unwired: 2 in, 2 out]
            n736 = property on="WriteToFile" class="Bool (strict)"("Disabled"=w691) -> ()  [unwired: 2 in, 2 out]
            n737 = property on="SetCurrentB" class="Bool (strict)"("Disabled"=w691) -> ()  [unwired: 2 in, 2 out]
            n738 = property on="SetOutputOnB" class="Bool (strict)"("Disabled"=w691) -> ()  [unwired: 2 in, 2 out]
            n739 = property on="SetVoltageB" class="Bool (strict)"("Disabled"=w691) -> ()  [unwired: 2 in, 2 out]
            n740 = property on="SetOutputOffB" class="Bool (strict)"("Disabled"=w691) -> ()  [unwired: 2 in, 2 out]
            n741 = property on="SetVoltageAll" class="Bool (strict)"("Disabled"=w691) -> ()  [unwired: 2 in, 2 out]
            n742 = property on="SetCurrentAll" class="Bool (strict)"("Disabled"=w691) -> ()  [unwired: 2 in, 2 out]
            n743 = property on="DisconnectAll" class="Bool (strict)"("Disabled"=w691) -> ()  [unwired: 2 in, 2 out]
          }
        }
      }
      event "DeleteChannel": Value Change {
        n744 = event-data() -> ()  [unwired: 7 out]
        n745 = property on="List of channels" class="MCListbox (strict)"() -> ("Value"=w695:i32)  [unwired: 2 in, 2 out]
        n746 = flat-sequence {
          tunnel: [w704] -> w696
          tunnel: w695 -> [w704]
          tunnel: [w708] -> w703
          tunnel: [w706] -> w702
          tunnel: [w707] -> w701
          tunnel: w696 -> [w706]
          tunnel: [w714] -> w700
          tunnel: w703 -> [w714]
          tunnel: [w713] -> w699
          tunnel: w702 -> [w713]
          tunnel: w701 -> [w712]
          tunnel: [w712] -> w698
          tunnel: w700 -> [w719]
          tunnel: [w718] -> w697
          tunnel: w699 -> [w718]
          tunnel: w698 -> [w717]
          tunnel: [w716] -> w693
          tunnel: w697 -> [w721]
          tunnel: [w720] -> w694
          tunnel: w693 -> [w720]
          tunnel: w694 -> [w729]
          tunnel: [w729] -> w692
          frame #0 {
            w705 = u8 2 ("Disabled")
            n747 = property on="AddChannel" class="Bool (strict)"("Disabled"=w705) -> ()  [unwired: 2 in, 2 out]
            n748 = property on="Set Output ON All" class="Bool (strict)"("Disabled"=w705) -> ()  [unwired: 2 in, 2 out]
            n749 = property on="ConnectAll" class="Bool (strict)"("Disabled"=w705) -> ()  [unwired: 2 in, 2 out]
            n750 = property on="DisconnectChannel" class="Bool (strict)"("Disabled"=w705) -> ()  [unwired: 2 in, 2 out]
            n751 = property on="ReadFromFile" class="Bool (strict)"("Disabled"=w705) -> ()  [unwired: 2 in, 2 out]
            n752 = property on="Quit" class="Bool (strict)"("Disabled"=w705) -> ()  [unwired: 2 in, 2 out]
            n753 = property on="ConnectChannel" class="Bool (strict)"("Disabled"=w705) -> ()  [unwired: 2 in, 2 out]
            n754 = property on="DeleteChannel" class="Bool (strict)"("Disabled"=w705) -> ()  [unwired: 2 in, 2 out]
            n755 = property on="WriteToFile" class="Bool (strict)"("Disabled"=w705) -> ()  [unwired: 2 in, 2 out]
            n756 = property on="SetCurrentB" class="Bool (strict)"("Disabled"=w705) -> ()  [unwired: 2 in, 2 out]
            n757 = property on="SetOutputOnB" class="Bool (strict)"("Disabled"=w705) -> ()  [unwired: 2 in, 2 out]
            n758 = property on="SetVoltageB" class="Bool (strict)"("Disabled"=w705) -> ()  [unwired: 2 in, 2 out]
            n759 = property on="SetOutputOffB" class="Bool (strict)"("Disabled"=w705) -> ()  [unwired: 2 in, 2 out]
            n760 = property on="SetVoltageAll" class="Bool (strict)"("Disabled"=w705) -> ()  [unwired: 2 in, 2 out]
            n761 = property on="SetCurrentAll" class="Bool (strict)"("Disabled"=w705) -> ()  [unwired: 2 in, 2 out]
            n762 = property on="DisconnectAll" class="Bool (strict)"("Disabled"=w705) -> ()  [unwired: 2 in, 2 out]
          }
          frame #1 {
            n763 = local read "Measure_VI"() -> (w710:refnum<vi>[])
            n764 = Index Array(array=w710, index=w706) -> (element=w708:refnum<vi>)
            n765 = invoke class="VI" method="Ctrl Val.Set"(reference=w708, "Control Name"="Connect", "Value"=FALSE ("OK Button")) -> (error out=w707:errorcluster)  [unwired: 2 in, 4 out]
          }
          frame #2 {
            n766 = Wait (ms)(milliseconds to wait=u32 1000) -> ()  [unwired: 1 out]
          }
          frame #3 {
            n767 = invoke class="VI" method="Abort VI"(reference=w719, error in=w717) -> (error out=w716:errorcluster)  [unwired: 1 in, 2 out]
          }
          frame #4 {
            w722 = 1 ("length")
            n768 = local read "Measure_VI"() -> (w728:refnum<vi>[])
            n769 = local read "ADRESS"() -> (w727:string[])
            n770 = local read "NAME"() -> (w723:string[])
            n771 = Delete From Array(array=w728, length=w722, index=w721) -> (array with subset deleted=w725:refnum<vi>[])  [unwired: 1 out]
            n772 = Delete From Array(array=w727, length=w722, index=w721) -> (array with subset deleted=w726:string[])  [unwired: 1 out]
            n773 = Delete From Array(array=w723, length=w722, index=w721) -> (array with subset deleted=w724:string[])  [unwired: 1 out]
            n774 = local write "ADRESS"(w726) -> ()
            n775 = local write "Measure_VI"(w725) -> ()
            n776 = local write "NAME"(w724) -> ()
          }
          frame #5 {
            w730 = u8 0 ("Disabled")
            n777 = local write "DeleteChannel"(FALSE ("DeleteChannel")) -> ()
            n778 = property on="AddChannel" class="Bool (strict)"("Disabled"=w730) -> ()  [unwired: 2 in, 2 out]
            n779 = property on="DisconnectChannel" class="Bool (strict)"("Disabled"=w730) -> ()  [unwired: 2 in, 2 out]
            n780 = property on="ReadFromFile" class="Bool (strict)"("Disabled"=w730) -> ()  [unwired: 2 in, 2 out]
            n781 = property on="ConnectChannel" class="Bool (strict)"("Disabled"=w730) -> ()  [unwired: 2 in, 2 out]
            n782 = property on="Quit" class="Bool (strict)"("Disabled"=w730) -> ()  [unwired: 2 in, 2 out]
            n783 = property on="DeleteChannel" class="Bool (strict)"("Disabled"=w730) -> ()  [unwired: 2 in, 2 out]
            n784 = property on="WriteToFile" class="Bool (strict)"("Disabled"=w730) -> ()  [unwired: 2 in, 2 out]
            n785 = property on="Set Output ON All" class="Bool (strict)"("Disabled"=w730) -> ()  [unwired: 2 in, 2 out]
            n786 = property on="SetCurrentB" class="Bool (strict)"("Disabled"=w730) -> ()  [unwired: 2 in, 2 out]
            n787 = property on="ConnectAll" class="Bool (strict)"("Disabled"=w730) -> ()  [unwired: 2 in, 2 out]
            n788 = property on="SetOutputOnB" class="Bool (strict)"("Disabled"=w730) -> ()  [unwired: 2 in, 2 out]
            n789 = property on="SetVoltageB" class="Bool (strict)"("Disabled"=w730) -> ()  [unwired: 2 in, 2 out]
            n790 = property on="SetOutputOffB" class="Bool (strict)"("Disabled"=w730) -> ()  [unwired: 2 in, 2 out]
            n791 = property on="SetVoltageAll" class="Bool (strict)"("Disabled"=w730) -> ()  [unwired: 2 in, 2 out]
            n792 = property on="SetCurrentAll" class="Bool (strict)"("Disabled"=w730) -> ()  [unwired: 2 in, 2 out]
            n793 = property on="DisconnectAll" class="Bool (strict)"("Disabled"=w730) -> ()  [unwired: 2 in, 2 out]
          }
        }
      }
    }
    n794 = call <vilib>:"General Error Handler.vi"("type of dialog (OK msg:1)"=u8 0 ("Disabled"), "error in (no error)"=w200) -> ()  [unwired: 14 out]
    n795 = Wait Until Next ms Multiple(millisecond multiple=u32 20) -> ()  [unwired: 1 out]
  }
  n796 = property on="Set Output ON All" class="Bool (strict)"("Disabled"=w21) -> (error out=w15:errorcluster)  [unwired: 2 in, 1 out]
  n797 = property on="SetCurrentAll" class="Bool (strict)"("Disabled"=w21) -> ()  [unwired: 2 in, 2 out]
  n798 = property on="AddChannel" class="Bool (strict)"("Disabled"=w21) -> ()  [unwired: 2 in, 2 out]
  n799 = property on="AddChannel" class="Bool (strict)"("Disabled"=u8 0) -> ()  [unwired: 2 in, 2 out]
  n800 = local write "текущий ист."(u8 0 ("текущий ист.")) -> ()
  n801 = local write "WriteToFile"(w23) -> ()
  n802 = local write "DisconnectChannel"(w23) -> ()
  n803 = local write "ConnectChannel"(w23) -> ()
  n804 = local write "SetCurrentB"(w23) -> ()
  n805 = local write "ReadFromFile"(w23) -> ()
  n806 = local write "AddChannel"(w23) -> ()
  n807 = local write "Quit"(w23) -> ()
  n808 = local write "SetCurrentAll"(w23) -> ()
  n809 = local write "SetVoltageAll"(w23) -> ()
  n810 = local write "DeleteChannel"(w23) -> ()
  n811 = local write "SetVoltageB"(w23) -> ()
  n812 = local write "SetOutputOnB"(w6) -> ()
  n813 = local write "ConnectAll"(w6) -> ()
  n814 = local write "SetOutputOffB"(w6) -> ()
  n815 = local write "DisconnectAll"(w6) -> ()
  n816 = disable-structure shown="Disabled" {
    frame Disabled {
      n817 = call <vilib>:"Application Directory.vi"() -> ("Application Directory"=w749:path)
      n818 = Build Path(base path=w749, name or relative path="BuvConfig.dat") -> (appended path=w746:path)
      n819 = Open/Create/Replace File(file path (use dialog)=w746, operation (0:open)=T2."open") -> (refnum out=w744:refnum<file>, error out=w745:errorcluster)  [unwired: 4 in, 1 out]
      n820 = Read from Text File(file (use dialog)=w744, error in=w745) -> (text=w741:string, error out=w736:errorcluster)  [unwired: 2 in, 2 out]
      n821 = Match Pattern(string=w741, regular expression="Z" ("string")) -> (before substring=w740:string, after substring=w737:string)  [unwired: 1 in, 2 out]
      n822 = Scan From String(input string=w737, error in=w736) -> (error out=w733:errorcluster, output 1=w738:dbl)  [unwired: 3 in, 2 out]
      n823 = local write item#-1(w738) -> ()
      n824 = Scan From String(input string=w740, error in=w733, default 1=u16 0 ("default value 1")) -> (error out=w735:errorcluster, output 1=w743:u16)  [unwired: 2 in, 2 out]
      n825 = local write item#-1(w743) -> ()
      n826 = case shown="No Error" w735 {
        selector: w735 -> [w793 w795]
        tunnel: [TRUE ("LoadPhase") FALSE ("LoadPhase")] -> w734
        tunnel: [w793 w795] -> w732
        frame No Error {
        }
        frame Error {
        }
      }
      "LoadPhase" <- w734
      n827 = while {
        tunnel: w732 -> [w750]
        stop <- FALSE stop-if-true
        n828 = flat-sequence {
          tunnel: [w763] -> w758
          tunnel: [w762] -> w757
          tunnel: w750 -> [w761]
          tunnel: w758 -> [w770]
          tunnel: w757 -> [w769]
          tunnel: [w768] -> w756
          tunnel: [w767] -> w755
          tunnel: w756 -> [w781]
          tunnel: [w780] -> w754
          tunnel: w755 -> [w779]
          tunnel: [w778] -> w753
          tunnel: w754 -> [w784]
          tunnel: w753 -> [w783]
          tunnel: [_] -> w752
          tunnel: [_] -> w751
          tunnel: w752 -> [w791]
          tunnel: w751 -> [w788]
          frame #0 {
            n829 = TCP Open Connection(address="172.16.21.81", remote port or service name=u16 4001, timeout ms (60000)=1000, error in (no error)=w761) -> (connection ID=w762:refnum<k5>, error out=w763:errorcluster)  [unwired: 1 in]
            "Buv con ID" <- w762
          }
          frame #1 {
            n830 = case shown="No Error" w770 {
              selector: w770 -> [w771 w777]
              tunnel: w769 -> [w772 w776]
              tunnel: [_ w777] -> w768
              tunnel: [_ w776] -> w767
              frame No Error {
                n831 = local read item#-1() -> (w774)
                n832 = Or(y=w774) -> (x .or. y?=w773:bool)  [unwired: 1 in]
                n833 = case shown="True" w773 {
                  tunnel: w772 -> [_ _]
                  tunnel: w771 -> [_ _]
                  frame False {
                  }
                  frame True {
                    # "Установка опорного напряжения"
                    n834 = local write item#-1(FALSE ("LoadPhase")) -> ()
                  }
                }
              }
              frame Error {
              }
            }
          }
          frame #2 {
          }
          frame #3 {
            n835 = case shown="Error" w784 {
              selector: w784 -> [_ w786]
              tunnel: w783 -> [_ w785]
              tunnel: [_ "*"] -> _
              tunnel: [_ w786] -> w782
              tunnel: [_ w785] -> _
              frame No Error {
              }
              frame Error {
              }
            }
          }
          frame #4 {
            n836 = case shown="Error" w788 {
              frame No Error {
              }
              frame Error {
                w792 = TRUE ("LoadPhase")
                n837 = local write "LoadPhase"(w792) -> ()
                n838 = local write item#-1(w792) -> ()
              }
            }
            n839 = TCP Close Connection(connection ID=w791) -> (error out=w790:errorcluster)  [unwired: 2 in, 1 out]
            n840 = call <vilib>:"General Error Handler.vi"("type of dialog (OK msg:1)"=0 ("milliseconds to wait"), "error in (no error)"=w790) -> ()  [unwired: 9 in, 5 out]
          }
        }
        n841 = Wait Until Next ms Multiple(millisecond multiple=u32 70) -> ()  [unwired: 1 out]
      }
    }
    frame Enabled {
    }
  }
  n842 = property on="DisconnectAll" class="Bool (strict)"(error in=w15, "Disabled"=w21) -> (error out=w14:errorcluster)  [unwired: 1 in, 1 out]
  n843 = property on="DisconnectChannel" class="Bool (strict)"("Disabled"=w21) -> (error out=w20:errorcluster)  [unwired: 2 in, 1 out]
  n844 = property on="WriteToFile" class="Bool (strict)"(error in=w14, "Disabled"=w21) -> (error out=w13:errorcluster)  [unwired: 1 in, 1 out]
  n845 = property on="SetCurrentB" class="Bool (strict)"(error in=w13, "Disabled"=w21) -> (error out=w12:errorcluster)  [unwired: 1 in, 1 out]
  n846 = property on="ConnectAll" class="Bool (strict)"(error in=w20, "Disabled"=w21) -> (error out=w19:errorcluster)  [unwired: 1 in, 1 out]
  n847 = property on="Quit" class="Bool (strict)"(error in=w12, "Disabled"=w21) -> (error out=w11:errorcluster)  [unwired: 1 in, 1 out]
  n848 = property on="ReadFromFile" class="Bool (strict)"(error in=w19, "Disabled"=w21) -> (error out=w18:errorcluster)  [unwired: 1 in, 1 out]
  n849 = property on="SetOutputOnB" class="Bool (strict)"(error in=w11, "Disabled"=w21) -> (error out=w10:errorcluster)  [unwired: 1 in, 1 out]
  n850 = property on="ConnectChannel" class="Bool (strict)"(error in=w18, "Disabled"=w21) -> (error out=w17:errorcluster)  [unwired: 1 in, 1 out]
  n851 = property on="SetVoltageB" class="Bool (strict)"(error in=w10, "Disabled"=w21) -> (error out=w9:errorcluster)  [unwired: 1 in, 1 out]
  n852 = property on="SetOutputOffB" class="Bool (strict)"(error in=w9, "Disabled"=w21) -> ()  [unwired: 1 in, 2 out]
  n853 = property on="DeleteChannel" class="Bool (strict)"(error in=w17, "Disabled"=w21) -> (error out=w16:errorcluster)  [unwired: 1 in, 1 out]
  n854 = property on="SetVoltageAll" class="Bool (strict)"(error in=w16, "Disabled"=w21) -> ()  [unwired: 1 in, 2 out]
  n855 = event shown="[0] \"Quit\": Value Change" {
    selector: _ -> [_]
    dyn-events: _ -> [_]
    timeout: _ -> [_]
    event "Quit": Value Change {
      n856 = event-data() -> ()  [unwired: 1 in, 1 out]
      n857 = flat-sequence {
        frame #0 {
          w803 = T3 0 items=["no dialog", "OK message", "continue or stop message", "OK message + warnings", "continue/stop + warnings"] ("type of dialog (OK msg:1)")
          n858 = local read "BuvCtrlVI_VIRef"() -> (w800:refnum<vi>[])
          n859 = local read "Measure_VI"() -> (w798:refnum<vi>[])
          n860 = Array Size(array=w800) -> (size(s)=w802:i32)
          n861 = Array Size(array=w798) -> (size(s)=w799:i32)
          n862 = for {
            N: w802 -> [_]
            tunnel: [w838] -> w801 mode=indexing
            tunnel: w800 -> [w837]
            i -> [w839]
            n863 = Index Array(array=w837, index=w839) -> (element=w831:refnum<vi>)
            n864 = To Variant(anything=TRUE ("ConnectChannel")) -> (Variant=w834:variant)
            n865 = invoke on="Invoke Node" class="VI" method="Ctrl Val.Set"(reference=w831, "Control Name"="TCP disconnect", "Value"=w834) -> (reference out=w833:refnum<vi>, error out=w832:errorcluster)  [unwired: 2 in, 3 out]
            n866 = flat-sequence {
              tunnel: [w842] -> w830
              tunnel: w833 -> [w842]
              tunnel: [w841] -> w829
              tunnel: w832 -> [w841]
              frame #0 {
                n867 = Wait (ms)(milliseconds to wait=u32 100) -> ()  [unwired: 1 out]
              }
            }
            n868 = invoke class="VI" method="Abort VI"(reference=w830, error in=w829) -> (error out=w838:errorcluster)  [unwired: 1 in, 2 out]
          }
          n869 = for {
            N: w799 -> [_]
            tunnel: [w815] -> w797 mode=indexing
            tunnel: w798 -> [w814]
            i -> [w816]
            n870 = Index Array(array=w814, index=w816) -> (element=w808:refnum<vi>)
            n871 = To Variant(anything=TRUE ("ConnectChannel")) -> (Variant=w811:variant)
            n872 = invoke on="Invoke Node" class="VI" method="Ctrl Val.Set"(reference=w808, "Control Name"="TCP disconnect", "Value"=w811) -> (reference out=w810:refnum<vi>, error out=w809:errorcluster)  [unwired: 2 in, 3 out]
            n873 = flat-sequence {
              tunnel: [w819] -> w807
              tunnel: w810 -> [w819]
              tunnel: [w818] -> w806
              tunnel: w809 -> [w818]
              frame #0 {
                n874 = Wait (ms)(milliseconds to wait=u32 100) -> ()  [unwired: 1 out]
              }
            }
            n875 = invoke class="VI" method="Abort VI"(reference=w807, error in=w806) -> (error out=w815:errorcluster)  [unwired: 1 in, 2 out]
          }
          n876 = disable-structure shown="Disabled" {
            disable-tunnel: [w821 _] -> w805
            frame Disabled {
              n877 = local read "Measure_VI"() -> (w820:refnum<vi>[])
              n878 = Array Size(array=w820) -> (size(s)=w822:i32)
              n879 = for {
                N: w822 -> [_]
                tunnel: [w824] -> w821 mode=indexing
                tunnel: w820 -> [w823]
                i -> [w825]
                n880 = Index Array(array=w823, index=w825) -> (element=w827:refnum<vi>)
                n881 = invoke class="VI" method="Ctrl Val.Set"(reference=w827, "Control Name"="Connect", "Value"=FALSE ("OK Button")) -> (error out=w824:errorcluster)  [unwired: 2 in, 4 out]
              }
            }
            frame Enabled {
            }
          }
          n882 = Merge Errors(w797, w805, w801) -> (w804:errorcluster)
          n883 = call <vilib>:"General Error Handler.vi"("type of dialog (OK msg:1)"=w803, "error in (no error)"=w804) -> ()  [unwired: 9 in, 5 out]
        }
        frame #1 {
          n884 = Wait (ms)(milliseconds to wait=u32 200) -> ()  [unwired: 1 out]
        }
        frame #2 {
          n885 = Stop(stop? (T)=TRUE) -> ()
        }
      }
    }
  }
  n886 = while {
    stop <- FALSE stop-if-true
    w848 = T3 0 items=["no dialog", "OK message", "continue or stop message", "OK message + warnings", "continue/stop + warnings"] ("type of dialog (OK msg:1)")
    # "БУВы"
    n887 = event shown="[3] \"ReadFromFile Buv\": Value Change" {
      selector: _ -> [_ _ _ _ _]
      dyn-events: _ -> [_ _ _ _ _]
      timeout: _ -> [_ _ _ _ _]
      tunnel: [w856 w898 w922 w938 w1006] -> w847
      event #0 (no event record) {
        # "ВКЛ/ВЫКЛ силовую часть выбранного БУВа, уст. напрядения"
        n888 = event-data() -> ("id"=w850, "ВКЛ."=w860, "ВЫКЛ."=w859, "ВКЛ."=w858, "ВЫКЛ."=w857)  [unwired: 1 in, 4 out]
        n889 = Not Equal?() -> (x != y?=w855:bool)  [unwired: 2 in]
        n890 = case shown="11" {
          selector: _ -> [w868 w870 w871 w872 w873 w874 w875 w876 w877 w878 w879 w880]
          tunnel: [w869 _ _ _ _ _ _ _ _ _ _ _] -> _
          tunnel: [w868 w870 w871 w872 w873 w874 w875 w876 w877 w878 w879 w880] -> w851
          frame 0, Default {
            n891 = local read item#-1() -> (w869)
          }
          frame 1 {
            n892 = local read item#-1() -> ()  [unwired: 1 out]
          }
          frame 2 {
            n893 = local read item#-1() -> ()  [unwired: 1 out]
          }
          frame 3 {
            n894 = local read item#-1() -> ()  [unwired: 1 out]
          }
          frame 4 {
            n895 = local read item#-1() -> ()  [unwired: 1 out]
          }
          frame 5 {
            n896 = local read item#-1() -> ()  [unwired: 1 out]
          }
          frame 6 {
            n897 = local read item#-1() -> ()  [unwired: 1 out]
          }
          frame 7 {
            n898 = local read item#-1() -> ()  [unwired: 1 out]
          }
          frame 8 {
            n899 = local read item#-1() -> ()  [unwired: 1 out]
          }
          frame 9 {
            n900 = local read item#-1() -> ()  [unwired: 1 out]
          }
          frame 10 {
            n901 = local read item#-1() -> ()  [unwired: 1 out]
          }
          frame 11 {
            n902 = local read item#-1() -> ()  [unwired: 1 out]
          }
        }
        n903 = Bundle By Name("ВКЛ."=w858, "ВЫКЛ."=w857) -> (w853:cluster{})  [unwired: 1 in]
        n904 = local read "BuvCtrlVI_VIRef"() -> (w865:refnum<vi>[])
        n905 = Index Array(array=w865) -> (element=w852:refnum<vi>)  [unwired: 1 in]
        n906 = To Variant(anything=w860) -> (Variant=w867:variant)
        n907 = To Variant(anything=w859) -> (Variant=w863:variant)
        n908 = case shown="True" w855 {
          tunnel: w852 -> [_ w884]
          tunnel: [_ w883] -> w854
          tunnel: w850 -> [_ _]
          frame False {
          }
          frame True {
            n909 = Multiply(y=1.5) -> (x*y=w882:dbl)  [unwired: 1 in]
            n910 = To Variant() -> (Variant=w889:variant)  [unwired: 1 in]
            n911 = invoke class="VI" method="Ctrl Val.Set"(reference=w884, "Control Name"="SetVoltage", "Value"=w889) -> (reference out=w887:refnum<vi>, error out=w888:errorcluster)  [unwired: 2 in, 3 out]
            n912 = case shown="12" {
              selector: _ -> [_ _ _ _ _ _ _ _ _ _ _ _ _]
              tunnel: w882 -> [_ _ _ _ _ _ _ _ _ _ _ _ _]
              frame 0, Default {
                # "Уст. макс. знач. слайдера"
              }
              frame 1 {
              }
              frame 2 {
              }
              frame 3 {
              }
              frame 4 {
              }
              frame 5 {
              }
              frame 6 {
              }
              frame 7 {
              }
              frame 8 {
              }
              frame 9 {
              }
              frame 10 {
              }
              frame 11 {
              }
              frame 12 {
              }
            }
            n913 = To Variant(anything=TRUE ("ConnectChannel")) -> (Variant=w890:variant)
            n914 = invoke class="VI" method="Ctrl Val.Set"(reference=w887, error in=w888, "Control Name"="SetV", "Value"=w890) -> (error out=w883:errorcluster)  [unwired: 1 in, 4 out]
          }
        }
        n915 = case shown="9" w851 {
          tunnel: w853 -> [_ _ _ _ _ _ _ _ _ _ _ _]
          frame 0, Default {
            n916 = local read item#-1() -> ()  [unwired: 1 in]
          }
          frame 1 {
            n917 = local read item#-1() -> ()  [unwired: 1 in]
          }
          frame 2 {
            n918 = local read item#-1() -> ()  [unwired: 1 in]
          }
          frame 3 {
            n919 = local read item#-1() -> ()  [unwired: 1 in]
          }
          frame 4 {
            n920 = local read item#-1() -> ()  [unwired: 1 in]
          }
          frame 5 {
            n921 = local read item#-1() -> ()  [unwired: 1 in]
          }
          frame 6 {
            n922 = local read item#-1() -> ()  [unwired: 1 in]
          }
          frame 7 {
            n923 = local read item#-1() -> ()  [unwired: 1 in]
          }
          frame 8 {
            n924 = local read item#-1() -> ()  [unwired: 1 in]
          }
          frame 9 {
            n925 = local read item#-1() -> ()  [unwired: 1 in]
          }
          frame 10 {
            n926 = local read item#-1() -> ()  [unwired: 1 in]
          }
          frame 11 {
            n927 = local read item#-1() -> ()  [unwired: 1 in]
          }
        }
        n928 = invoke class="VI" method="Ctrl Val.Set"(reference=w852, "Control Name"="SetOutON", "Value"=w867) -> (error out=w862:errorcluster)  [unwired: 2 in, 4 out]
        n929 = invoke class="VI" method="Ctrl Val.Set"(reference=w852, "Control Name"="SetOutOFF", "Value"=w863) -> (error out=w861:errorcluster)  [unwired: 2 in, 4 out]
        n930 = Merge Errors(w854, w862, w861) -> (w856:errorcluster)
      }
      event "AddNewBuv": Value Change {
        n931 = event-data() -> ("OldVal"=w904:bool)  [unwired: 1 in]
        n932 = local write "AddNewBuv"(w904) -> ()
        n933 = local read "BuvCtrlVI_VIRef"() -> (w903:refnum<vi>[])
        n934 = local read "BuvNameArr"() -> (w901:string[])
        n935 = local read "Buv IP"() -> (w897:string[])
        n936 = call "AddNewBuv.vi"("Num of Buvs in"="Num of Buvs", "New BuV IP"="NewBuvIP", "Voltage"="0", "Name Arr IN"=w901, "New BuV name"="NewBuvName", "Buv IP arr"=w897, "BuvCtrlVI_VIRef"=w903) -> ("BuvCtrlVI_VIRefOut"=w902:refnum<vi>[], "Num of Buvs out"=w892:u8, "Name Out"=w899:string[], "Buv Ip Out"=w900:string[], "error out"=w898:errorcluster)  [unwired: 16 in]
        n937 = local write "BuvNameArr"(w899) -> ()
        n938 = local write "BuvCtrlVI_VIRef"(w902) -> ()
        n939 = local write "Num of Buvs"(w892) -> ()
        n940 = local write "Buv IP"(w900) -> ()
      }
      event "DeleteBuv": Value Change {
        n941 = event-data() -> ("OldVal"=w926:bool)  [unwired: 1 in]
        n942 = local read "Num of Buvs"() -> (w924:u8)
        n943 = local write "DeleteBuv"(w926) -> ()
        n944 = local read "BuvCtrlVI_VIRef"() -> (w925:refnum<vi>[])
        n945 = Decrement(x=w924) -> (x-1=w923:u8)
        n946 = Index Array(array=w925) -> (element=w920:refnum<vi>)  [unwired: 1 in]
        n947 = To Variant(anything=TRUE ("ConnectChannel")) -> (Variant=w918:variant)
        n948 = local write "Num of Buvs"(w923) -> ()
        n949 = invoke on="Invoke Node" class="VI" method="Ctrl Val.Set"(reference=w920, "Control Name"="TCP disconnect", "Value"=w918) -> (reference out=w916:refnum<vi>, error out=w914:errorcluster)  [unwired: 2 in, 3 out]
        n950 = flat-sequence {
          tunnel: [w929] -> w917
          tunnel: w916 -> [w929]
          tunnel: [w928] -> w915
          tunnel: w914 -> [w928]
          frame #0 {
            n951 = Wait (ms)(milliseconds to wait=u32 100) -> ()  [unwired: 1 out]
          }
        }
        n952 = invoke class="VI" method="Abort VI"(reference=w917, error in=w915) -> (error out=w922:errorcluster)  [unwired: 1 in, 2 out]
        n953 = local read "BuvCtrlVI_VIRef"() -> (w910:refnum<vi>[])
        n954 = local read "BuvNameArr"() -> (w909:string[])
        n955 = local read "Buv IP"() -> (w908:string[])
        n956 = Delete From Array(array=w910, length=1) -> (array with subset deleted=w907:refnum<vi>[])  [unwired: 1 in, 1 out]
        n957 = Delete From Array(array=w909, length=1) -> (array with subset deleted=w906:string[])  [unwired: 1 in, 1 out]
        n958 = Delete From Array(array=w908, length=1) -> (array with subset deleted=w905:string[])  [unwired: 1 in, 1 out]
        n959 = local write "BuvCtrlVI_VIRef"(w907) -> ()
        n960 = local write "BuvNameArr"(w906) -> ()
        n961 = local write "Buv IP"(w905) -> ()
      }
      event "ReadFromFile Buv": Value Change {
        n962 = event-data() -> ("OldVal"=w937:bool)  [unwired: 1 in]
        n963 = call "File Dialog2"("start path"=path "C:/", "prompt"="Укажите конфигурационный файл" ("prompt (Open existing file)"), "pattern (all files)"="*.dat", "pattern label"="Настройки ЛЖФ") -> ("selected path"=w935:path, "error out"=w932:errorcluster)  [unwired: 8 in, 2 out]
        n964 = Read from Text File(file (use dialog)=w935, count=-1, error in=w932) -> (text=w943:string[], cancelled=w939:bool, error out=w944:errorcluster)  [unwired: 2 out]
        n965 = Not(x=w939) -> (.not. x?=w941:bool)
        n966 = Not(x=w944) -> (.not. x?=w942:bool)
        n967 = And(x=w941, y=w942) -> (x .and. y?=w940:bool)
        n968 = local write "ReadFromFile Buv"(w937) -> ()
        n969 = case shown="True" w940 {
          tunnel: w943 -> [_ w952]
          tunnel: [w946 w950] -> w945
          tunnel: w944 -> [w947 w948]
          frame False {
            n970 = Build Array(w947) -> (w946:errorcluster[])
          }
          frame True {
            n971 = flat-sequence {
              tunnel: w952 -> [w955]
              tunnel: [w955] -> w951
              tunnel: [w954] -> w949
              tunnel: w948 -> [w954]
              tunnel: w951 -> [w960]
              tunnel: [w959] -> w950
              tunnel: w949 -> [w958]
              frame #0 {
                w956 = string[] [] ("Buv IP")
                n972 = local write "Num of Buvs"(u8 0 ("Num of Buvs")) -> ()
                "Buv IP" <- w956
                "BuvNameArr" <- w956
                "BuvCtrlVI_VIRef" <- refnum<vi>[] [] ("BuvCtrlVI_VIRef")
              }
              frame #1 {
                n973 = Index Array(array=w960, index=0) -> (element=w962:string)
                n974 = Decimal String To Number(string=w962) -> (number=w961:i32)  [unwired: 3 out]
                n975 = for {
                  N: w961 -> [_]
                  tunnel: w960 -> [w990]
                  tunnel: [w983] -> w959 mode=indexing
                  tunnel: w958 -> [w984]
                  i -> [w966]
                  # "Добавление нового БУВа"
                  n976 = Increment(x=w966) -> (x+1=w969:i32)
                  n977 = Index Array(array=w990, index=w969) -> (element=w973:string)
                  n978 = Spreadsheet String To Array(format string="%s", spreadsheet string=w973, array type (2D Dbl)=string[] [] ("GlobalInAdress")) -> (array=w979:string[])  [unwired: 1 out]
                  n979 = local read "BuvCtrlVI_VIRef"() -> (w989:refnum<vi>[])
                  n980 = local read "Buv IP"() -> (w982:string[])
                  n981 = local read "BuvNameArr"() -> (w981:string[])
                  n982 = local read "Num of Buvs"() -> (w980:u8)
                  n983 = Index Array "Name"(array=w979, index=0) -> (element=w970:string)
                  n984 = Index Array "IP"(array=w979, index=1) -> (element=w972:string)
                  n985 = Index Array "SetV"(array=w979, index=2) -> (element=w967:string)
                  n986 = call "AddNewBuv.vi"("Num of Buvs in"=w980, "New BuV IP"=w972, "Voltage"=w967, "error in"=w984, "Name Arr IN"=w981, "New BuV name"=w970, "Buv IP arr"=w982, "BuvCtrlVI_VIRef"=w989) -> ("BuvCtrlVI_VIRefOut"=w988:refnum<vi>[], "Num of Buvs out"=w971:u8, "Name Out"=w986:string[], "Buv Ip Out"=w987:string[], "error out"=w985:errorcluster)  [unwired: 15 in]
                  n987 = Scan From String(format string="%f", input string=w967) -> (error out=w965:errorcluster, output 1=w964:dbl)  [unwired: 3 in, 2 out]
                  n988 = local write "BuvCtrlVI_VIRef"(w988) -> ()
                  n989 = case "Уст. напряж. из файла" shown="0, Default" w966 {
                    tunnel: w965 -> [_ _ _ _ _ _ _ _ _ _ _ _ _]
                    tunnel: w964 -> [_ _ _ _ _ _ _ _ _ _ _ _ _]
                    frame 0, Default {
                    }
                    frame 1 {
                    }
                    frame 2 {
                    }
                    frame 3 {
                    }
                    frame 4 {
                    }
                    frame 5 {
                    }
                    frame 6 {
                    }
                    frame 7 {
                    }
                    frame 8 {
                    }
                    frame 9 {
                    }
                    frame 10 {
                    }
                    frame 11 {
                    }
                    frame 12 {
                    }
                  }
                  n990 = flat-sequence {
                    tunnel: [w991] -> w983
                    tunnel: w985 -> [w991]
                    frame #0 {
                      n991 = Wait (ms)(milliseconds to wait=u32 50) -> ()  [unwired: 1 out]
                    }
                  }
                  n992 = local write "BuvNameArr"(w986) -> ()
                  n993 = local write "Buv IP"(w987) -> ()
                  n994 = local write "Num of Buvs"(w971) -> ()
                }
              }
            }
          }
        }
        n995 = Merge Errors(w945) -> (w938:errorcluster)
      }
      event "WriteToFile Buv": Value Change {
        w993 = "Настройки ЛЖФ " ("default name")
        # "Запись конфигурации БУВов в файл"
        n996 = event-data() -> ("OldVal"=w1011:bool)  [unwired: 1 in]
        n997 = local read "BuvCtrlVI_VIRef"() -> (w1010:refnum<vi>[])
        n998 = local write "WriteToFile Buv"(w1011) -> ()
        n999 = Array Size(array=w1010) -> (size(s)=w1009:i32)
        n1000 = Number To Decimal String(number=w1009) -> (decimal integer string=w1001:string)  [unwired: 1 out]
        n1001 = for {
          N: w1009 -> [_]
          tunnel: [w1014] -> w1008 mode=indexing
          tunnel: [w1012] -> w999 mode=indexing
          i -> [w1018]
          w1016 = "\t"
          n1002 = local read "BuvCtrlVI_VIRef"() -> (w1022:refnum<vi>[])
          n1003 = Index Array(array=w1022, index=w1018) -> (element=w1021:refnum<vi>)
          n1004 = invoke class="VI" method="Ctrl Val.Get"(reference=w1021, "Control Name"="SetVstr") -> (error out=w1024:errorcluster, "Get Control Value Variant"=w1023:variant)  [unwired: 2 in, 2 out]
          n1005 = local read "BuvNameArr"() -> (w1026:string[])
          n1006 = local read "Buv IP"() -> (w1025:string[])
          n1007 = Index Array(array=w1026, index=w1018) -> (element=w1027:string)
          n1008 = Index Array(array=w1025, index=w1018) -> (element=w1017:string)
          n1009 = Variant To Data(error in=w1024, type="" ("Control Name"), Variant=w1023) -> (data=w1015:string, error out=w1014:errorcluster)
          n1010 = Concatenate Strings(w1027, w1016, w1017, w1016, w1015, "\r\n") -> (w1012:string)
        }
        n1011 = Merge Errors(w1008) -> (w1007:errorcluster)
        n1012 = call "File Dialog"("start path"=path "C:/", "prompt"="Укажите имя и директорию файла" ("prompt (Choose or enter file path)"), "default name"=w993, "pattern (all files)"="*.dat", "pattern label"=w993) -> ("selected path"=w998:path, "error out"=w997:errorcluster)  [unwired: 7 in, 2 out]
        n1013 = Concatenate Strings(w1001, "\r\n", w999) -> (w1000:string)
        n1014 = Write to Text File(file (use dialog)=w998, text=w1000, error in=w997) -> (refnum out=w1004:refnum<file>, error out=w1005:errorcluster)  [unwired: 2 out]
        n1015 = Close File(refnum=w1004, error in=w1005) -> (error out=w1003:errorcluster)  [unwired: 1 out]
        n1016 = Merge Errors(w1003, w1007) -> (w1006:errorcluster)
      }
    }
    n1017 = call <vilib>:"General Error Handler.vi"("type of dialog (OK msg:1)"=w848, "error in (no error)"=w847) -> ("message"=→"message event":string)  [unwired: 9 in, 4 out]
    n1018 = Wait Until Next ms Multiple(millisecond multiple=u32 10) -> ()  [unwired: 1 out]
  }
  n1019 = while {
    stop <- FALSE stop-if-true
    w1030 = string[] [] ("GlobalInAdress")
    w1041 = T3 0 items=["no dialog", "OK message", "continue or stop message", "OK message + warnings", "continue/stop + warnings"] ("type of dialog (OK msg:1)")
    # "БУВы. Обновление данных и вывод в таблицу"
    n1020 = local read "BuvCtrlVI_VIRef"() -> (w1044:refnum<vi>[])
    n1021 = Wait Until Next ms Multiple(millisecond multiple=u32 10) -> ()  [unwired: 1 out]
    n1022 = Array Size(array=w1044) -> (size(s)=w1036:i32)
    n1023 = for {
      N: w1036 -> [_]
      tunnel: w1044 -> [w1129]
      tunnel: [w1091] -> w1039 mode=indexing
      tunnel: [w1084] -> w1038 mode=indexing
      shift-right: [w1067] -> w1031
      shift-left: w1030 -> [w1066]
      shift-right: [w1063] -> w1029
      shift-left: w1030 -> [w1064]
      shift-right: [w1059] -> w1028
      shift-left: w1030 -> [w1061]
      i -> [w1050]
      n1024 = Index Array(array=w1129, index=w1050) -> (element=w1095:refnum<vi>)
      n1025 = invoke class="VI" method="Ctrl Val.Get"(reference=w1095, "Control Name"="ReadV") -> (error out=w1114:errorcluster, "Get Control Value Variant"=w1124:variant)  [unwired: 2 in, 2 out]
      n1026 = invoke class="VI" method="Ctrl Val.Get"(reference=w1095, "Control Name"="ReadI") -> (error out=w1113:errorcluster, "Get Control Value Variant"=w1126:variant)  [unwired: 2 in, 2 out]
      n1027 = invoke class="VI" method="Ctrl Val.Get"(reference=w1095, "Control Name"="SetVoltage") -> (error out=w1110:errorcluster, "Get Control Value Variant"=w1116:variant)  [unwired: 2 in, 2 out]
      n1028 = invoke class="VI" method="Ctrl Val.Get"(reference=w1095, "Control Name"="Active_num") -> (error out=w1111:errorcluster, "Get Control Value Variant"=w1119:variant)  [unwired: 2 in, 2 out]
      n1029 = invoke class="VI" method="Ctrl Val.Get"(reference=w1095, "Control Name"="status cluster") -> (error out=w1112:errorcluster, "Get Control Value Variant"=w1122:variant)  [unwired: 2 in, 2 out]
      n1030 = invoke class="VI" method="Ctrl Val.Get"(reference=w1095, "Control Name"="ErrMessage") -> (error out=w1099:errorcluster, "Get Control Value Variant"=w1098:variant)  [unwired: 2 in, 2 out]
      n1031 = Variant To Data(error in=w1114, type="" ("Control Name"), Variant=w1124) -> (data=w1065:string, error out=w1090:errorcluster)
      n1032 = Variant To Data(error in=w1113, type="" ("Control Name"), Variant=w1126) -> (data=w1060:string, error out=w1088:errorcluster)
      n1033 = Variant To Data(error in=w1110, type=0.0 ("Active_num"), Variant=w1116) -> (data=w1101:dbl, error out=w1100:errorcluster)
      n1034 = Variant To Data(error in=w1112, type=cluster{bool, bool, bool} {FALSE, FALSE, FALSE} ("status cluster"), Variant=w1122) -> (data=w1107:cluster{bool, bool, bool}, error out=w1086:errorcluster)
      n1035 = Variant To Data(error in=w1099, type="" ("Control Name"), Variant=w1098) -> (data=w1091:string, error out=w1085:errorcluster)
      n1036 = Variant To Data(error in=w1111, type=i16 0 ("Active_num"), Variant=w1119) -> (data=w1105:i16, error out=w1087:errorcluster)
      n1037 = Format Into String(format string="%.1f", error in=w1100, w1101) -> (resulting string=w1062:string, error out=w1089:errorcluster)  [unwired: 1 in]
      n1038 = local read "Buv IP"() -> (w1083:string[])
      n1039 = local read "BuvNameArr"() -> (w1092:string[])
      n1040 = Merge Errors(w1090, w1089, w1088, w1087, w1086, w1085) -> (w1084:errorcluster)
      n1041 = Unbundle(w1107) -> (w1109:bool, w1108:bool)  [unwired: 1 out]
      n1042 = Boolean To (0,1)(Boolean=w1109) -> (0, 1=w1093:i16)
      n1043 = Boolean To (0,1)(Boolean=w1108) -> (0, 1=w1104:i16)
      n1044 = Index Array(array=w1083, index=w1050) -> ()  [unwired: 1 out]
      n1045 = Index Array(array=w1092, index=w1050) -> ()  [unwired: 1 out]
      n1046 = Build Array (concatenate)(w1066, w1065) -> (w1067:string[])
      n1047 = Build Array (concatenate)(w1064, w1062) -> (w1063:string[])
      n1048 = Build Array (concatenate)(w1061, w1060) -> (w1059:string[])
      n1049 = Number To Decimal String(number=w1093, width (-)=i16 1) -> (decimal integer string=w1069:string)
      n1050 = Number To Decimal String(number=w1104, width (-)=i16 1) -> (decimal integer string=w1068:string)
      n1051 = Number To Decimal String(number=w1105, width (-)=i16 1) -> (decimal integer string=w1070:string)
      n1052 = Equal?(x="1", y=w1069) -> (x = y?=w1082:bool)
      n1053 = Equal?(x="1", y=w1070) -> (x = y?=w1079:bool)
      n1054 = Equal?(x="1", y=w1068) -> (x = y?=w1073:bool)
      n1055 = Select(t=u32 4109312, s=w1079, f=u32 15329769) -> (s? t:f=w1053:u32)
      n1056 = Select(t=u32 4109312, s=w1082, f=u32 15329769) -> (s? t:f=w1056:u32)
      n1057 = Select(t=u32 16711680, s=w1073, f=u32 16448250) -> (s? t:f=w1051:u32)
      n1058 = Bundle(w1050, "milliseconds to wait"=6) -> (w1054:cluster{i32, "milliseconds to wait":i32})  [unwired: 1 in]
      n1059 = Bundle(w1050, "milliseconds to wait"=5) -> (w1057:cluster{i32, "milliseconds to wait":i32})  [unwired: 1 in]
      n1060 = Bundle(w1050, "milliseconds to wait"=7) -> (w1049:cluster{i32, "milliseconds to wait":i32})  [unwired: 1 in]
      n1061 = property on="List of LU buw" class="MCListbox (strict)"("ActiveCell"=w1054, "CellBG"=w1053) -> ()  [unwired: 2 in, 2 out]
      n1062 = property on="List of LU buw" class="MCListbox (strict)"("ActiveCell"=w1057, "CellBG"=w1056) -> ()  [unwired: 2 in, 2 out]
      n1063 = property on="List of LU buw" class="MCListbox (strict)"("ActiveCell"=w1049, "CellBG"=w1051) -> ()  [unwired: 2 in, 2 out]
    }
    "Error BuvVIctrl" <- w1039
    n1064 = Merge Errors(w1038) -> (w1037:errorcluster)  [unwired: 1 in]
    n1065 = local read "Buv IP"() -> (w1032:string[])
    n1066 = local read "BuvNameArr"() -> (w1033:string[])
    n1067 = call <vilib>:"General Error Handler.vi"("type of dialog (OK msg:1)"=w1041, "error in (no error)"=w1037) -> ("message"=→"message upd":string)  [unwired: 9 in, 4 out]
    n1068 = Build Array(w1033, w1032, w1031, w1028, w1029) -> (w1035:string[][])
    n1069 = case shown="True" {
      selector: _ -> [_ _]
      tunnel: [T1."Disabled and Grayed Out" ("Disabled") T1."Enabled" ("Disabled")] -> _
      tunnel: [T1."Enabled" ("Disabled") T1."Disabled and Grayed Out" ("Disabled")] -> _
      frame False {
      }
      frame True {
      }
    }
    n1070 = Transpose 2D Array(2D array=w1035) -> (transposed array=w1034:string[][])
    n1071 = property on="List of LU buw" class="MCListbox (strict)"("ItemNames"=w1034) -> ()  [unwired: 2 in, 2 out]
  }
  n1072 = for "инициализация цветов и размера ячеек табл." {
    N: 50 -> [_]
    i -> [w1133]
    # "Линзы пост. тока"
    n1073 = flat-sequence {
      tunnel: w1133 -> [w1138]
      tunnel: [w1138] -> w1132
      tunnel: w1132 -> [w1177]
      tunnel: [w1177] -> w1131
      tunnel: w1131 -> [w1190]
      frame #0 {
        w1134 = "Application font" ("Font Name")
        n1074 = Bundle(w1138, 4) -> (w1150:cluster{i32, i32})  [unwired: 1 in]
        n1075 = property on="active" class="MCListbox (strict)"("ActiveCell"=w1150, "Height"=u32 35 ("Active Cell:Cell Size:Height"), "CellFontSize"=u16 28 ("Size")) -> ()  [unwired: 2 in, 2 out]
        n1076 = Bundle(w1138, 0) -> (w1161:cluster{i32, i32})  [unwired: 1 in]
        n1077 = Bundle(w1138, 2) -> (w1137:cluster{i32, i32})  [unwired: 1 in]
        n1078 = Bundle(w1138, 3) -> (w1151:cluster{i32, i32})  [unwired: 1 in]
        n1079 = Bundle(w1138, 1) -> (w1160:cluster{i32, i32})  [unwired: 1 in]
        n1080 = Bundle(w1138, 6) -> (w1136:cluster{i32, i32})  [unwired: 1 in]
        n1081 = Bundle(w1138, 5) -> (w1135:cluster{i32, i32})  [unwired: 1 in]
        n1082 = property on="active" class="MCListbox (strict)"("ActiveCell"=w1161, "Height"=u32 35 ("Active Cell:Cell Size:Height"), "CellFontSize"=u16 28 ("Size"), "CellFontName"=w1134) -> ()  [unwired: 2 in, 2 out]
        n1083 = property on="active" class="MCListbox (strict)"("ActiveCell"=w1137, "Height"=u32 35 ("Active Cell:Cell Size:Height"), "CellFontSize"=u16 28 ("Size"), "CellFontName"=w1134) -> ()  [unwired: 2 in, 2 out]
        n1084 = property on="active" class="MCListbox (strict)"("ActiveCell"=w1151, "Height"=u32 35 ("Active Cell:Cell Size:Height"), "CellFontSize"=u16 28 ("Size"), "CellFontName"=w1134) -> ()  [unwired: 2 in, 2 out]
        n1085 = property on="active" class="MCListbox (strict)"("ActiveCell"=w1160, "Height"=u32 35 ("Active Cell:Cell Size:Height"), "CellFontSize"=u16 28 ("Size"), "CellFontName"=w1134) -> ()  [unwired: 2 in, 2 out]
        n1086 = property on="active" class="MCListbox (strict)"("ActiveCell"=w1136, "Height"=u32 35 ("Active Cell:Cell Size:Height"), "CellFontSize"=u16 28 ("Size"), "CellFontName"=w1134) -> ()  [unwired: 2 in, 2 out]
        n1087 = property on="active" class="MCListbox (strict)"("ActiveCell"=w1135, "Height"=u32 35 ("Active Cell:Cell Size:Height"), "CellFontSize"=u16 28 ("Size"), "CellFontName"=w1134) -> ()  [unwired: 2 in, 2 out]
      }
      frame #1 {
        w1173 = T4 {"Font Name"="Application font", "Size"=28, "Bold"=FALSE, "Italic"=FALSE, "Underline"=FALSE, "Strikeout"=FALSE, "Color"=6908265} ("Active Cell:Cell Font")
        w1168 = T4 {"Font Name"="Application font", "Size"=30, "Bold"=TRUE, "Italic"=FALSE, "Underline"=FALSE, "Strikeout"=FALSE, "Color"=2263842} ("Active Cell:Cell Font")
        n1088 = Bundle(w1177, 3) -> (w1164:cluster{i32, i32})  [unwired: 1 in]
        n1089 = Bundle(w1177, 2) -> (w1167:cluster{i32, i32})  [unwired: 1 in]
        n1090 = Bundle(w1177, 0) -> (w1175:cluster{i32, i32})  [unwired: 1 in]
        n1091 = Bundle(w1177, 5) -> (w1171:cluster{i32, i32})  [unwired: 1 in]
        n1092 = Bundle(w1177, 4) -> (w1170:cluster{i32, i32})  [unwired: 1 in]
        n1093 = property on="active" class="MCListbox (strict)"("ActiveCell"=w1164, "CellFont"=w1168) -> ()  [unwired: 2 in, 2 out]
        n1094 = property on="active" class="MCListbox (strict)"("ActiveCell"=w1167, "CellFont"=w1168) -> ()  [unwired: 2 in, 2 out]
        n1095 = property on="active" class="MCListbox (strict)"("ActiveCell"=w1175, "CellFont"=T4 {"Font Name"="Application font", "Size"=28, "Bold"=FALSE, "Italic"=FALSE, "Underline"=FALSE, "Strikeout"=FALSE, "Color"=0} ("Active Cell:Cell Font")) -> ()  [unwired: 2 in, 2 out]
        n1096 = property on="active" class="MCListbox (strict)"("ActiveCell"=w1171, "CellFont"=w1173) -> ()  [unwired: 2 in, 2 out]
        n1097 = property on="active" class="MCListbox (strict)"("ActiveCell"=w1170, "CellFont"=w1173) -> ()  [unwired: 2 in, 2 out]
      }
      frame #2 {
        w1189 = T4 {"Font Name"="Application font", "Size"=28, "Bold"=FALSE, "Italic"=FALSE, "Underline"=FALSE, "Strikeout"=FALSE, "Color"=0} ("Active Cell:Cell Font")
        n1098 = Bundle(w1190, 6) -> (w1184:cluster{i32, i32})  [unwired: 1 in]
        n1099 = Bundle(w1190, 8) -> (w1185:cluster{i32, i32})  [unwired: 1 in]
        n1100 = Bundle(w1190, 7) -> (w1186:cluster{i32, i32})  [unwired: 1 in]
        n1101 = property on="active" class="MCListbox (strict)"("ActiveCell"=w1184, "CellBG"=u32 16777225) -> (error out=w1183:errorcluster)  [unwired: 2 in, 1 out]
        n1102 = property on="error" class="MCListbox (strict)"("ActiveCell"=w1185, "CellBG"=u32 16777225) -> ()  [unwired: 2 in, 2 out]
        n1103 = property on="out" class="MCListbox (strict)"("ActiveCell"=w1186, "CellBG"=u32 16777225) -> (error out=w1187:errorcluster)  [unwired: 2 in, 1 out]
        n1104 = property on="active" class="MCListbox (strict)"(error in=w1183, "ActiveCell"=w1184, "CellFont"=w1189) -> ()  [unwired: 1 in, 2 out]
        n1105 = property on="active" class="MCListbox (strict)"(error in=w1187, "ActiveCell"=w1186, "CellFont"=w1189) -> ()  [unwired: 1 in, 2 out]
      }
    }
  }
  n1106 = Build Array(w2, w2, w2, w2, w2, w2, w2, w2) -> (w3:string[][])
  n1107 = local write "BuvCtrlVI_VIRef"(refnum<vi>[] [] ("BuvCtrlVI_VIRef")) -> ()
  n1108 = Transpose 2D Array(2D array=w3) -> (transposed array=w4:string[][])
  n1109 = local write "BuvNameArr"(w5) -> ()
  n1110 = local write "Buv IP"(w5) -> ()
  n1111 = property on="List of channels" class="MCListbox (strict)"("ItemNames"=w4) -> ()  [unwired: 2 in, 2 out]
  "Measure_VI" <- refnum<vi>[] []
  "ADRESS" <- string[] [] ("GlobalInAdress")
  "NAME" <- string[] [] ("GlobalInAdress")
  "CURRENTSET" <- dbl[] [] ("GlobalInAdress")
